vi "4Pi Quadrant Phase Extractor.vi"(7 "Calling VI Ref":refnum<vi>) -> ()   [LabVIEW 2016]
uses:
  <vilib>/vision/Image Controls.llb/IMAQ Image.ctl
  Hardware Configuration/Hardware Configuration Controls/Device Type.ctl
  Hardware Configuration/Hardware Configuration Controls/Device Function.ctl
  Device Library/Cameras/Hamamatsu/Orca Flash/Orca Flash Controls/Orca Flash Actions.ctl
  Device Library/Stages/Stages Controls/Stage Actions.ctl
  Device Library/Cameras/Camera Controls/Camera IMAQ Key Info.ctl
  Device Library/Stages/Stages Controls/Stage Status.ctl
  Display Module/Display Module Custom Controls/ROI Descriptor.ctl
  <vilib>/gmath/NumericalOptimization/Nonlinear Curve Fit LM formula string.vi
  <vilib>/Utility/file.llb/Write Delimited Spreadsheet (DBL).vi
  <vilib>/vision/NI_Vision_Development_Module.lvlib
  <resource>/objmgr/IMAQImage.rc
  <vilib>/gmath/NI_Gmath.lvlib
panel:
  in  "Overlay Plot":bool
  out "Overlay Plot Graph":cluster{dbl[], dbl[]}[](graph)
  in  "Z Stack":bool
  in  "Save Data":bool
  in  "Velocity (µm/s)":dbl
  in  "Position (µm)":dbl
  in  "Scan Range (µm)":dbl
  in  "Fit 04":bool
  in  "Fit 03":bool
  in  "Fit 02":bool
  in  "Fit 01":bool
  in  "Initial Guess Image 04":T1={"Offset"=100.0, "Amplitude"=50.0, "Wavelength"=15.0, "Phase"=1.0}
  in  "Initial Guess Image 03":T1={"Offset"=100.0, "Amplitude"=50.0, "Wavelength"=15.0, "Phase"=1.0}
  in  "Initial Guess Image 02":T1={"Offset"=100.0, "Amplitude"=50.0, "Wavelength"=15.0, "Phase"=1.0}
  in  "Initial Guess Image 01":T1={"Offset"=100.0, "Amplitude"=50.0, "Wavelength"=15.0, "Phase"=1.0}
  in  "Run Scan":bool
  out "ROI Plot 04":cluster{dbl[], dbl[]}[](graph)
  in  "Interference Image 04":i32(ring) items=["Quad 01", "Quad 02", "Quad 03", "Quad 04"]
  out "ROI Plot 03":cluster{dbl[], dbl[]}[](graph)
  in  "Interference Image 03":i32(ring) items=["Quad 01", "Quad 02", "Quad 03", "Quad 04"]
  out "ROI Plot 02":cluster{dbl[], dbl[]}[](graph)
  in  "Interference Image 02":i32(ring) items=["Quad 01", "Quad 02", "Quad 03", "Quad 04"]
  out "ROI Plot 01":cluster{dbl[], dbl[]}[](graph)
  in  "Interference Image 01":i32(ring) items=["Quad 01", "Quad 02", "Quad 03", "Quad 04"]
  in  "Quit":bool
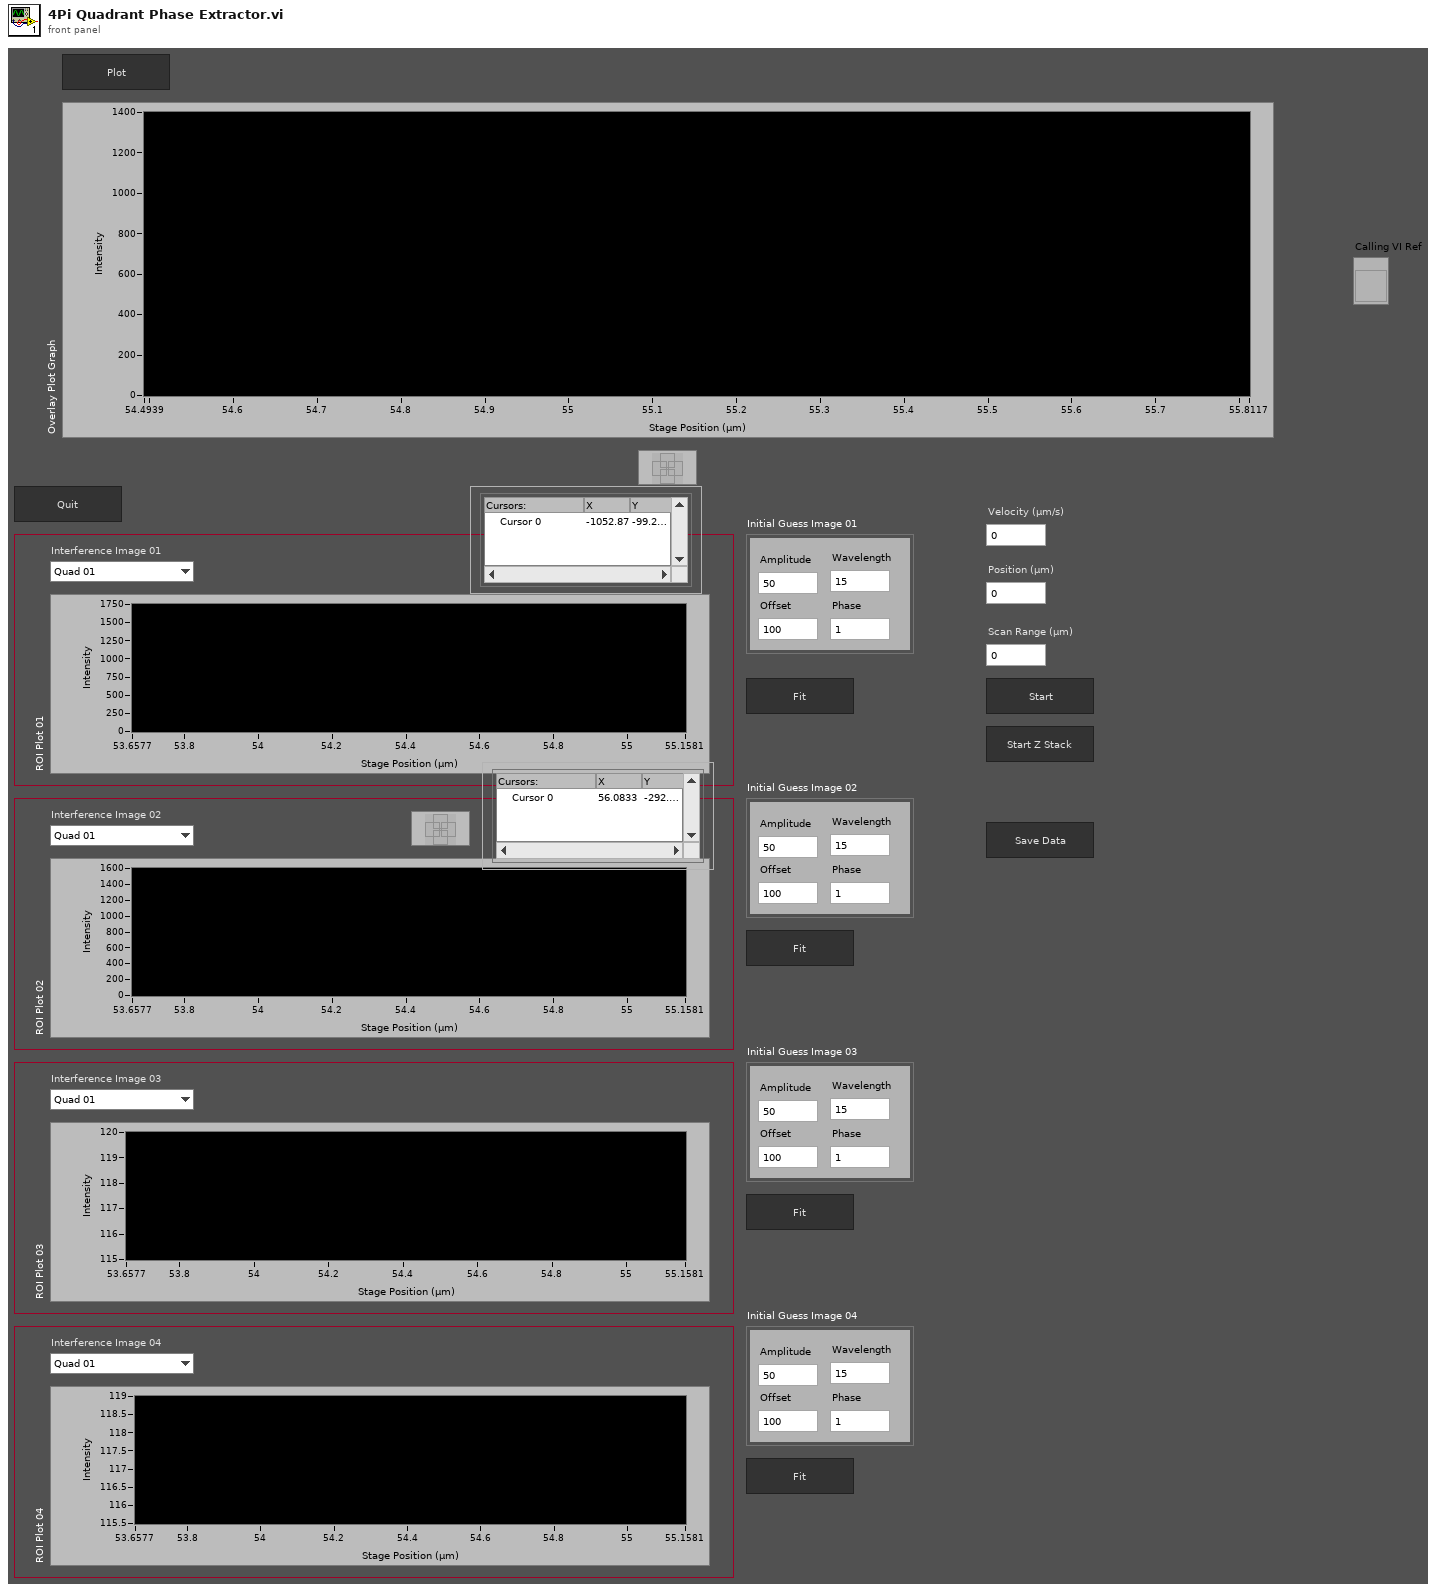
[diagram p1: front panel]
types:
  T1 = cluster{"Offset":dbl, "Amplitude":dbl, "Wavelength":dbl, "Phase":dbl}
  T2 = typedef "Device Function.ctl" = enum16{"Primary", "Secondary", "Overview", "Wide Field Drift Correction", "642 nm Excitation", "560 nm Excitation", "546 nm Excitation", "488 nm Excitation", "405 nm Excitation", "Objective Drift Correction", "Objective XY", "Objective Z", "Sample XY", "Sample Coarse Z", "Sample Z", "4Pi Lower", "4Pi Upper", "Adj Cavity"}
  T3 = typedef "Device Type.ctl" = enum16{"AOTF", "Camera", "Deformable Mirror", "Laser", "Shutter", "Stage"}
  T4 = typedef "Image Type" = u32
  T5 = typedef "Orca Flash Actions.ctl" = enum16{"IDLE", "PREVIEW", "RECORD", "Record Settings", "SETPARAM", "GETPARAM", "SETROI", "GETROI", "PROGRESSIVE MODE", "AREA MODE", "STATUS", "QUIT"}
  T6 = typedef "IMAQ Image.ctl" = refnum<image>
  T7 = typedef "Stage Actions.ctl" = enum16{"Get Position", "MVR", "MOVE", "HALT", "ONTARGET", "ERROR", "REFERENCE", "INIT", "VELOCITY", "STATUS", "EXIT", "HOME", "ZEROPOS", "NANOPOS", "ANALOG", "QUIT"}
  T8 = typedef "Camera IMAQ Key Info.ctl" = cluster{"Frame":u32, "Sensor Height":i32, "Sensor Width":i32, "ROI Height":i32, "ROI Width":i32, "ROI Enable?":bool, "Bit per Pixel":u8}
  T9 = typedef "Stage Status.ctl" = enum16{"Error", "Abort", "Busy", "On Target"}
  T10 = typedef "ROI Descriptor.ctl" = cluster{"Global Rectangle":i32[], "Contours":cluster{"Contour Type":u32, "ROI Type":u32, "Points":i32[]}[]}
  T11 = cluster{"model":string, "Parameters":string[], "x":string}
  T12 = cluster{"Mean Value":sgl, "Standard Variation":sgl, "Minimal Value":sgl, "Maximal Value":sgl, "Area (calibrated)":sgl, "Area (pixels)":u32, "%":sgl, "Calibration Valid":bool}
  T13 = cluster{"Numeric":dbl, "Numeric":dbl, "Numeric":dbl, "Numeric":dbl}
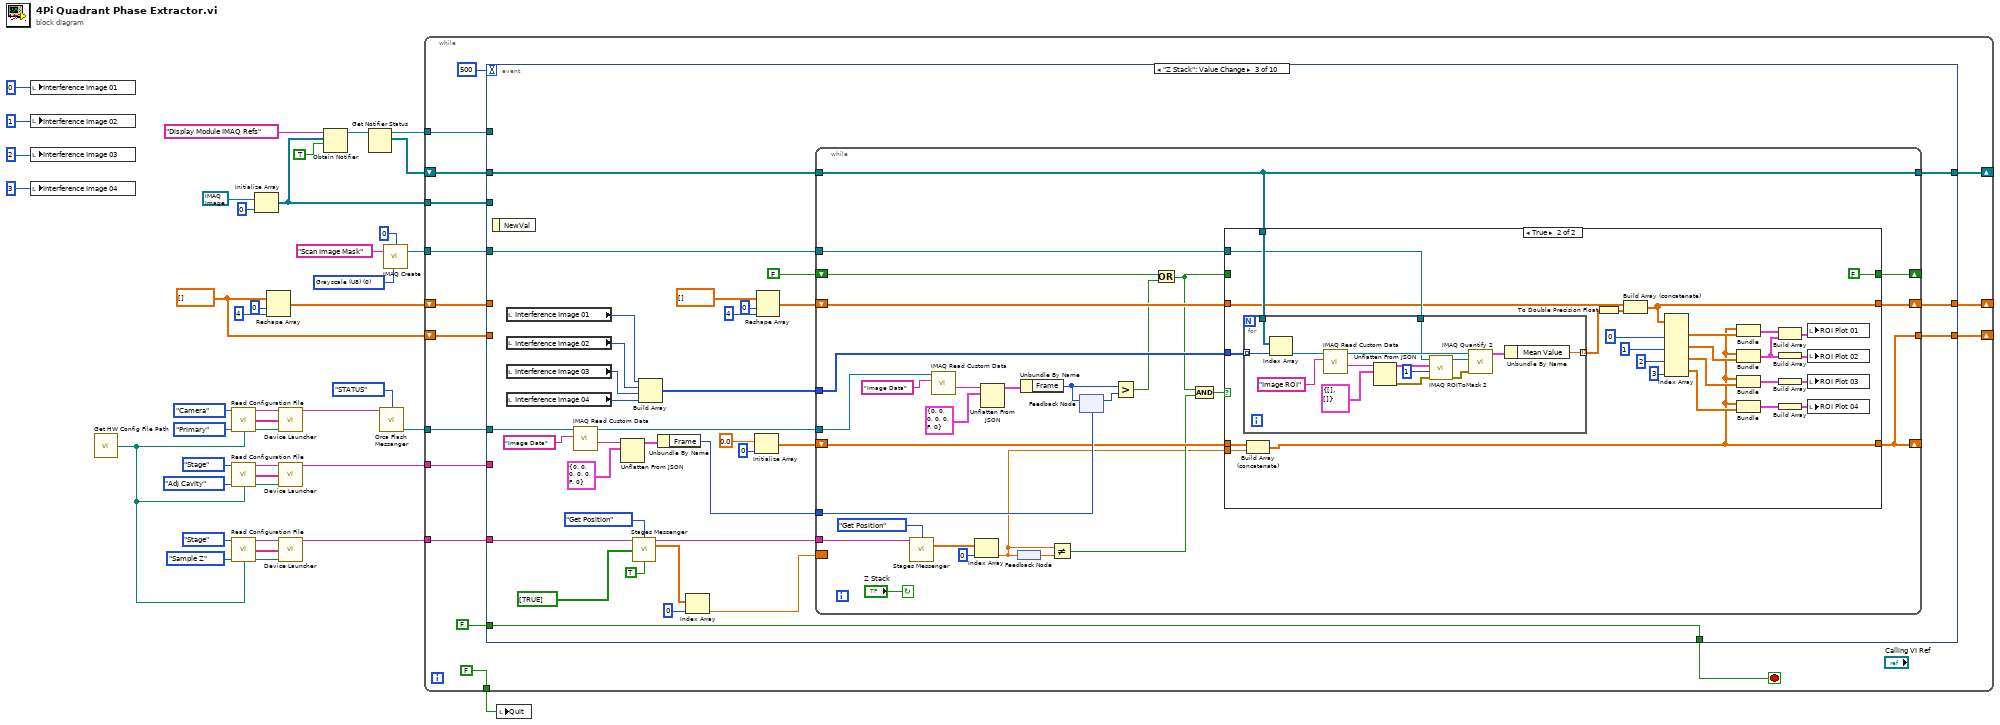
[diagram p0: block diagram]
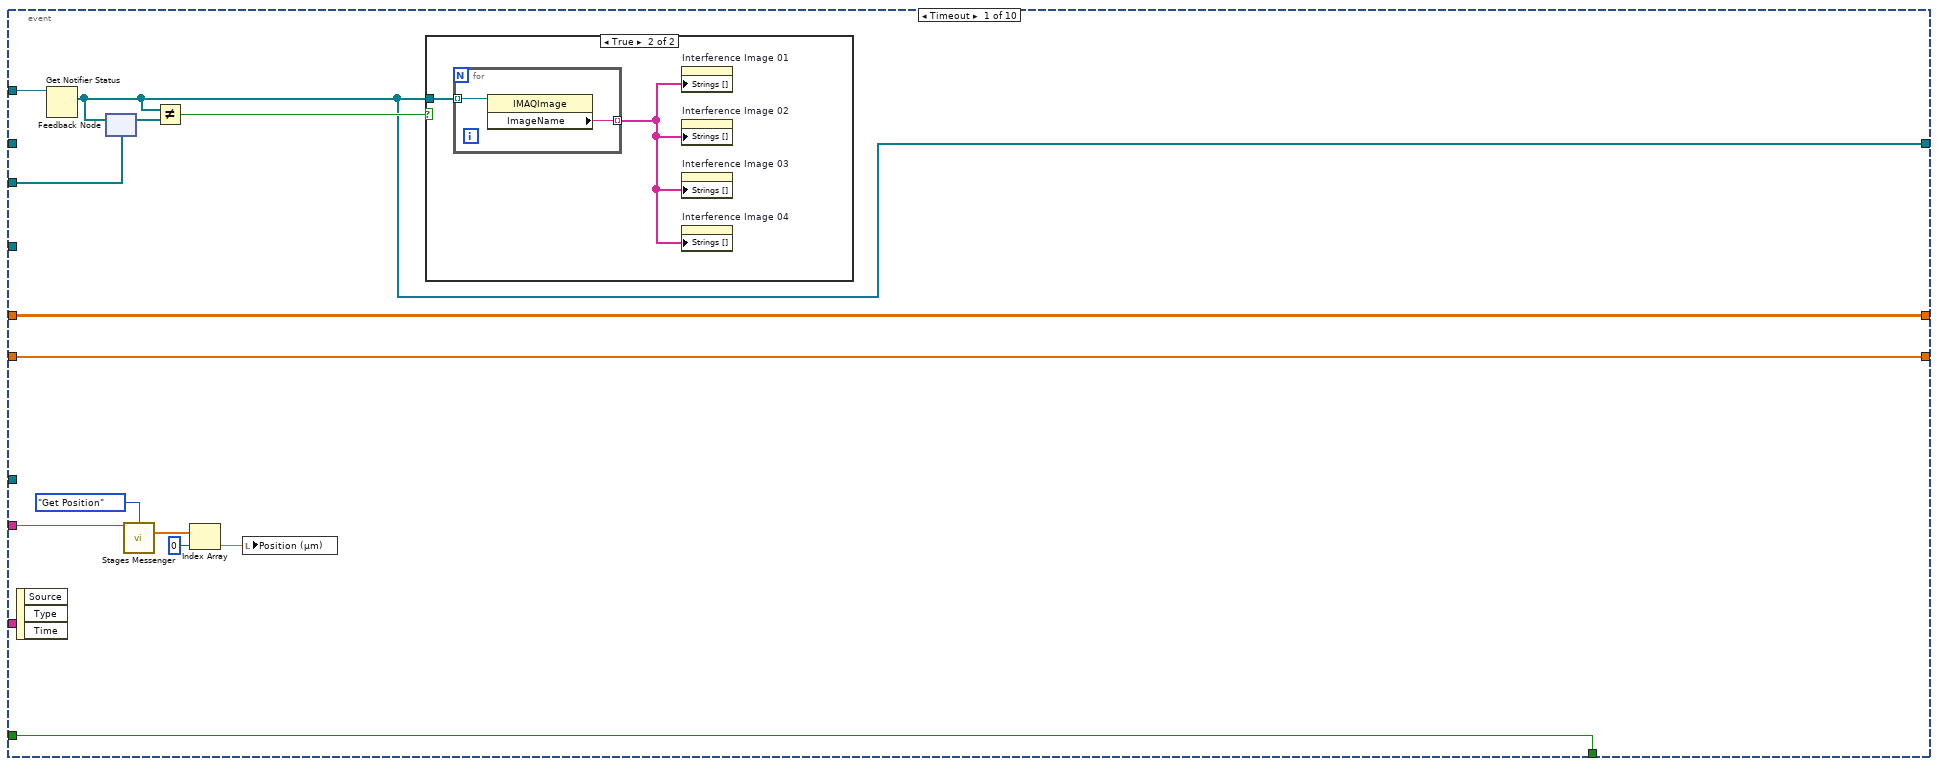
[diagram p2: hidden frame]
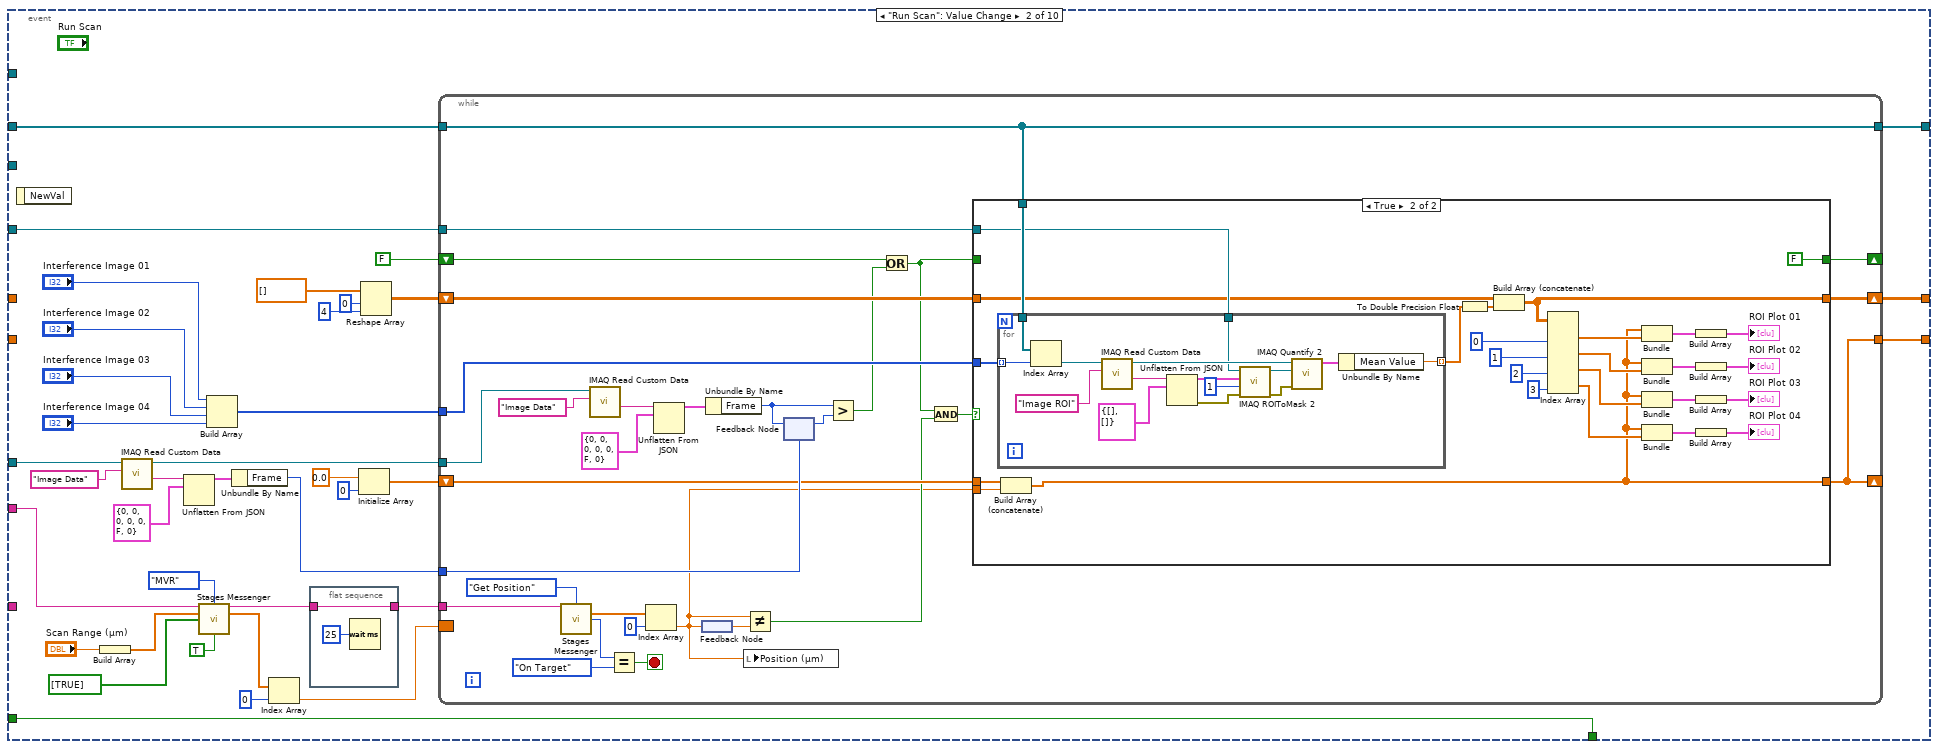
[diagram p4: hidden frame]
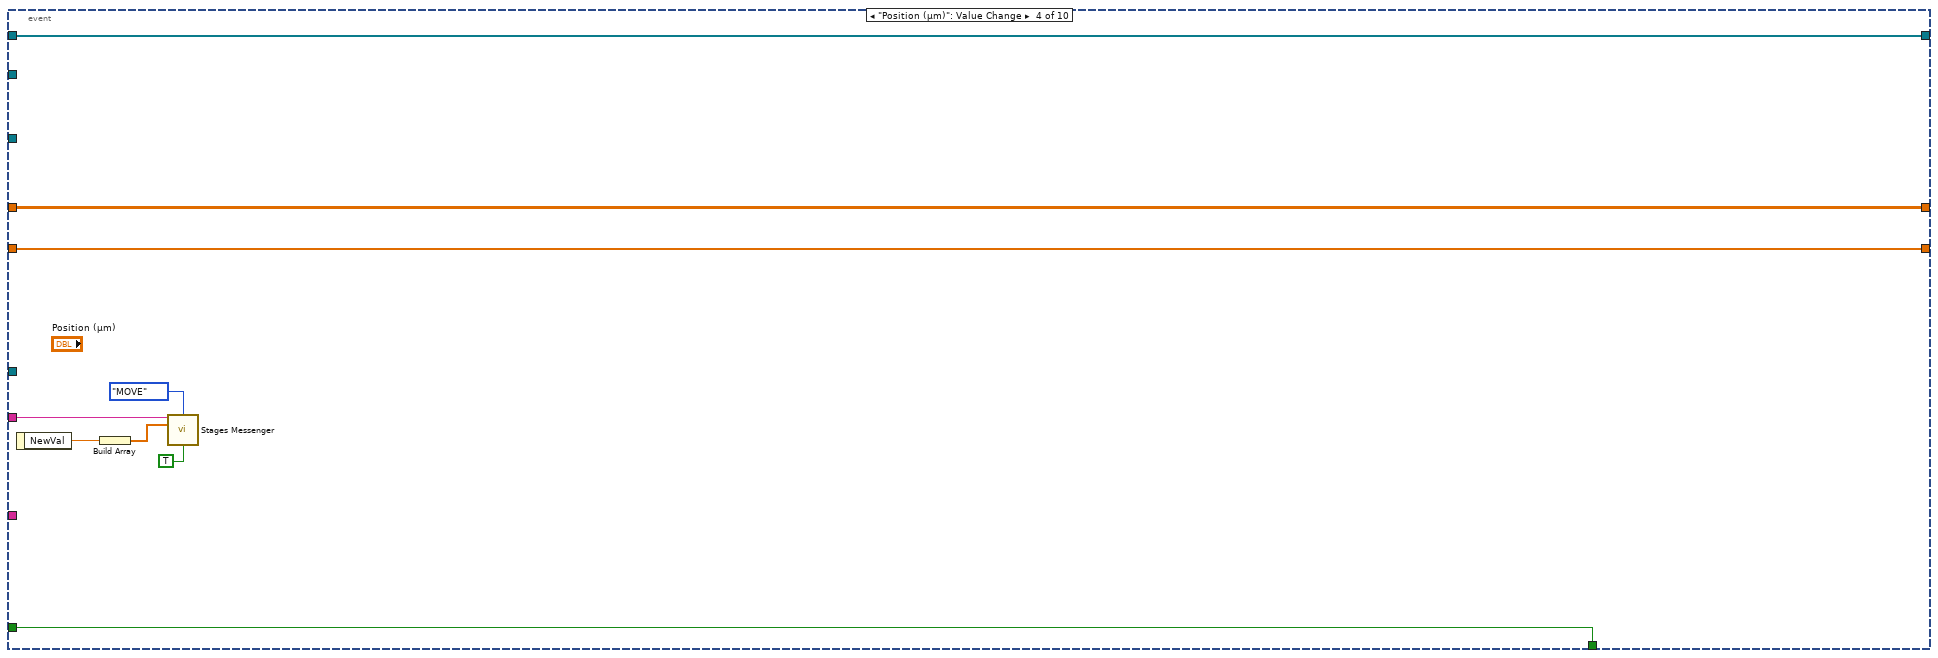
[diagram p7: hidden frame]
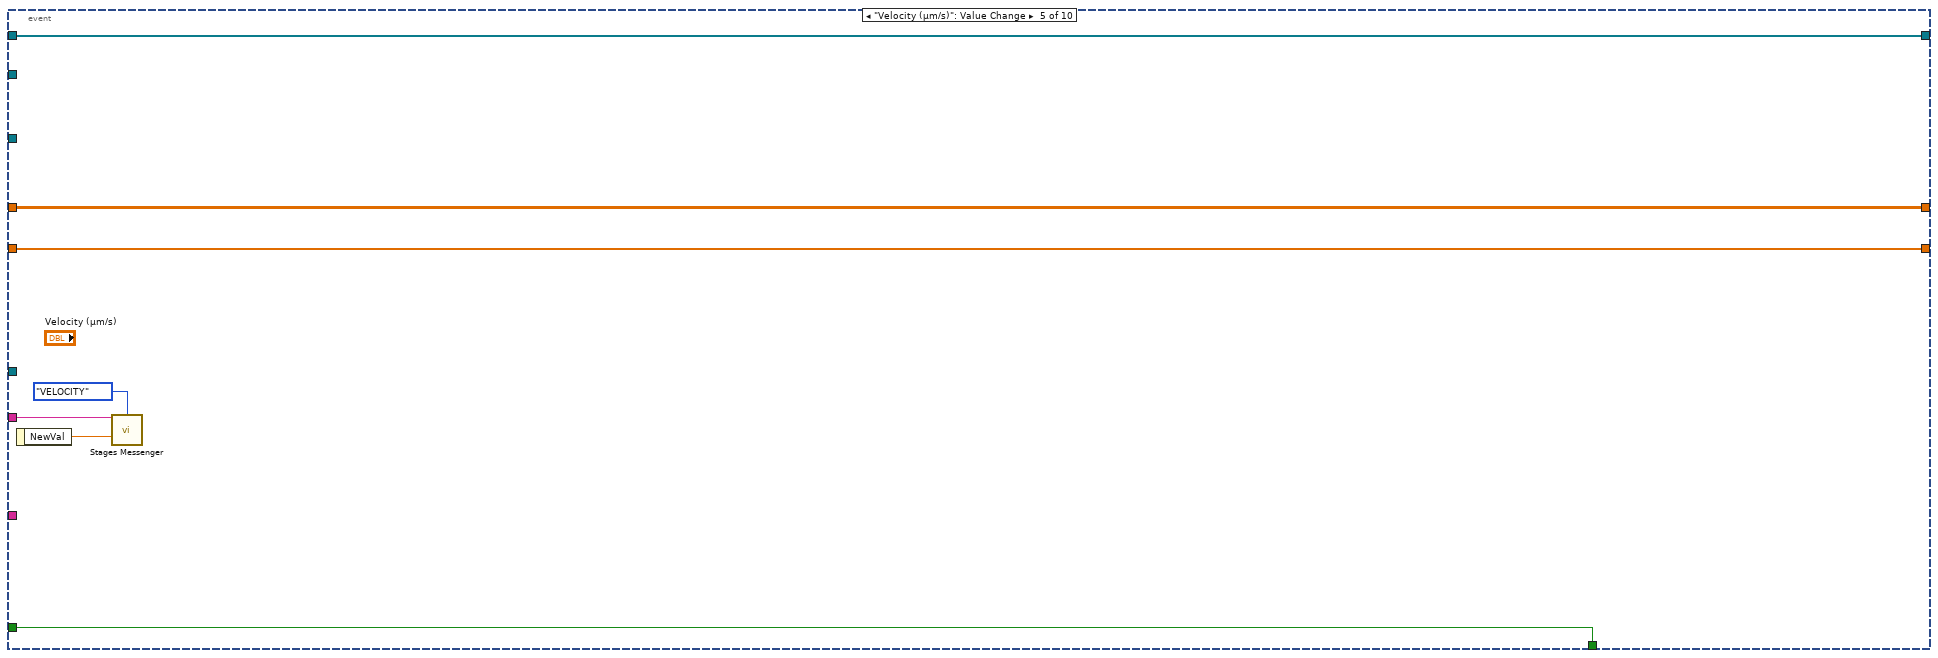
[diagram p8: hidden frame]
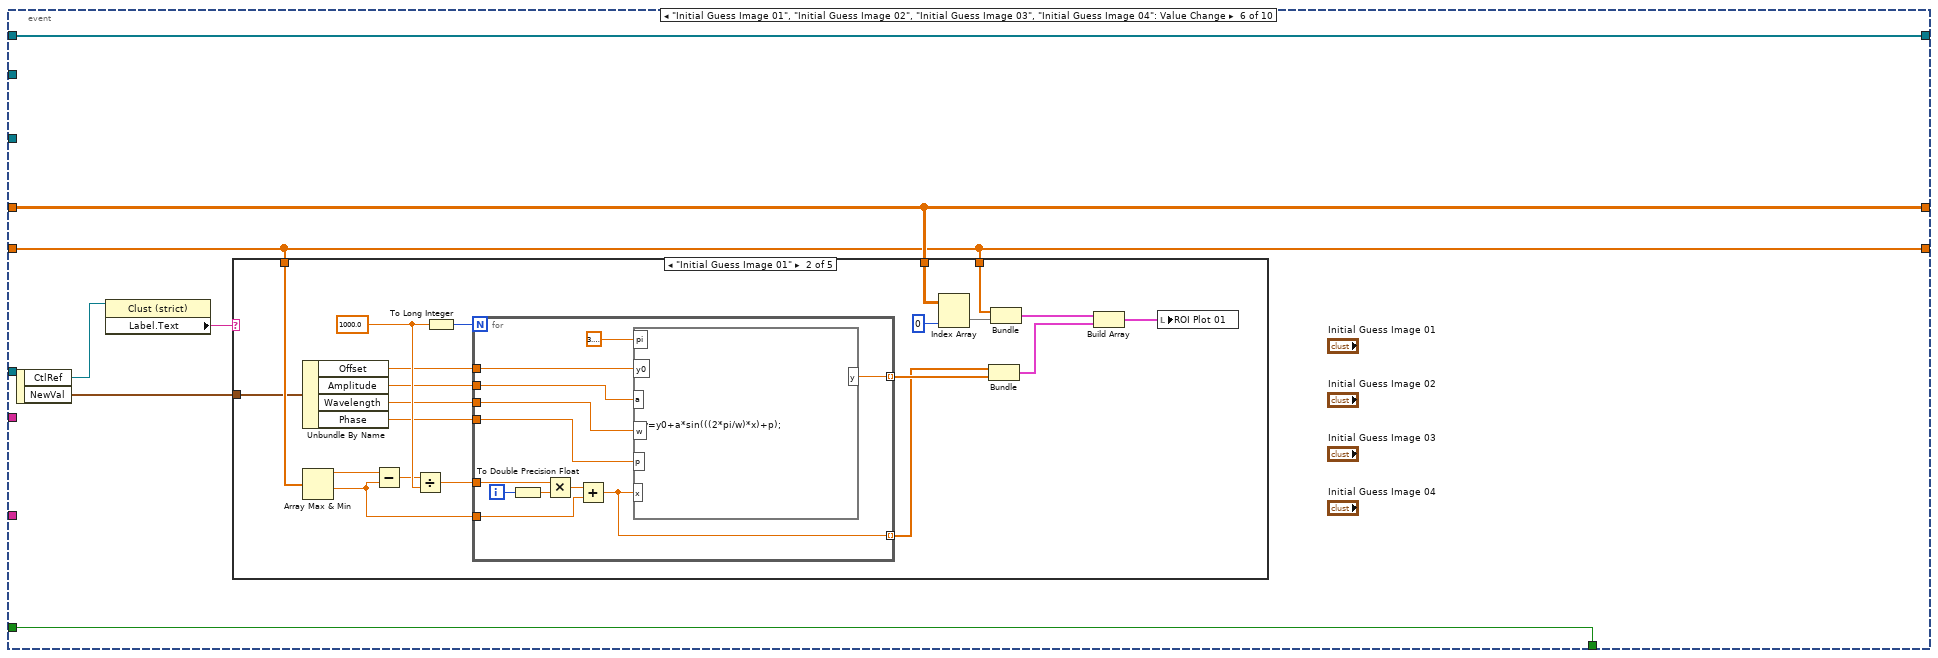
[diagram p9: hidden frame]
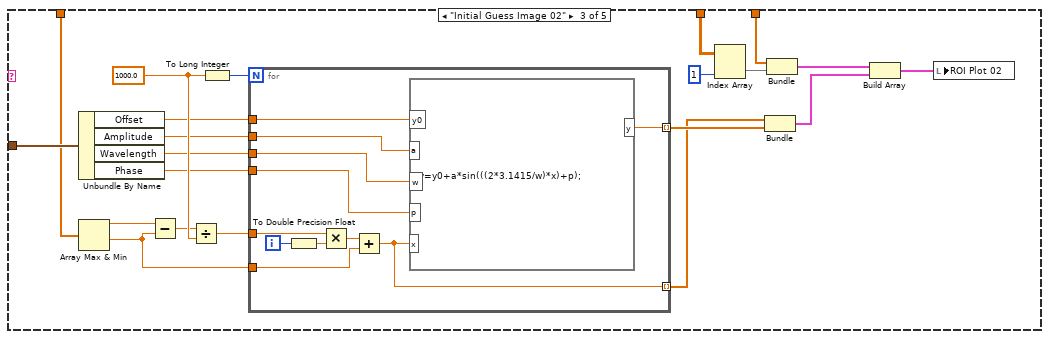
[diagram p11: hidden frame]
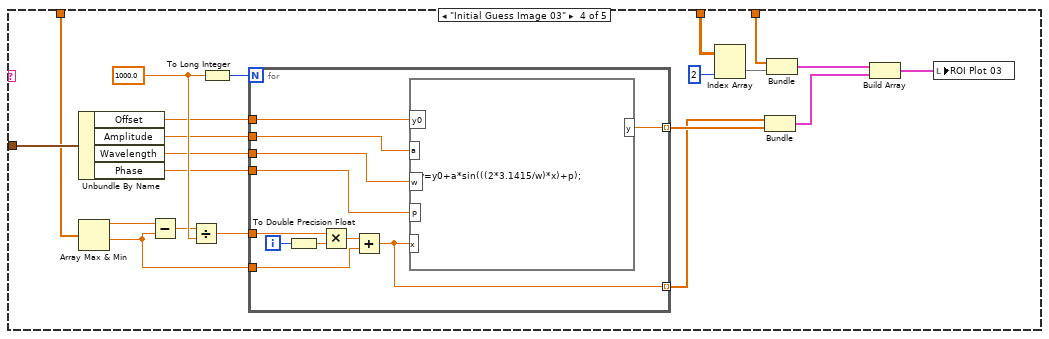
[diagram p12: hidden frame]
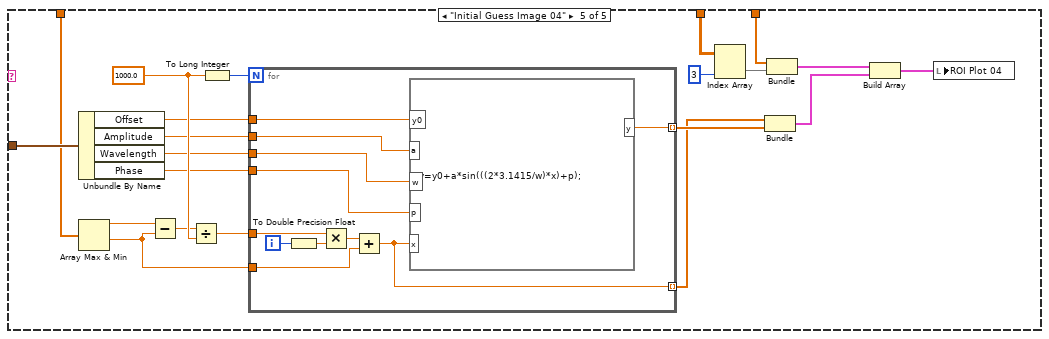
[diagram p13: hidden frame]
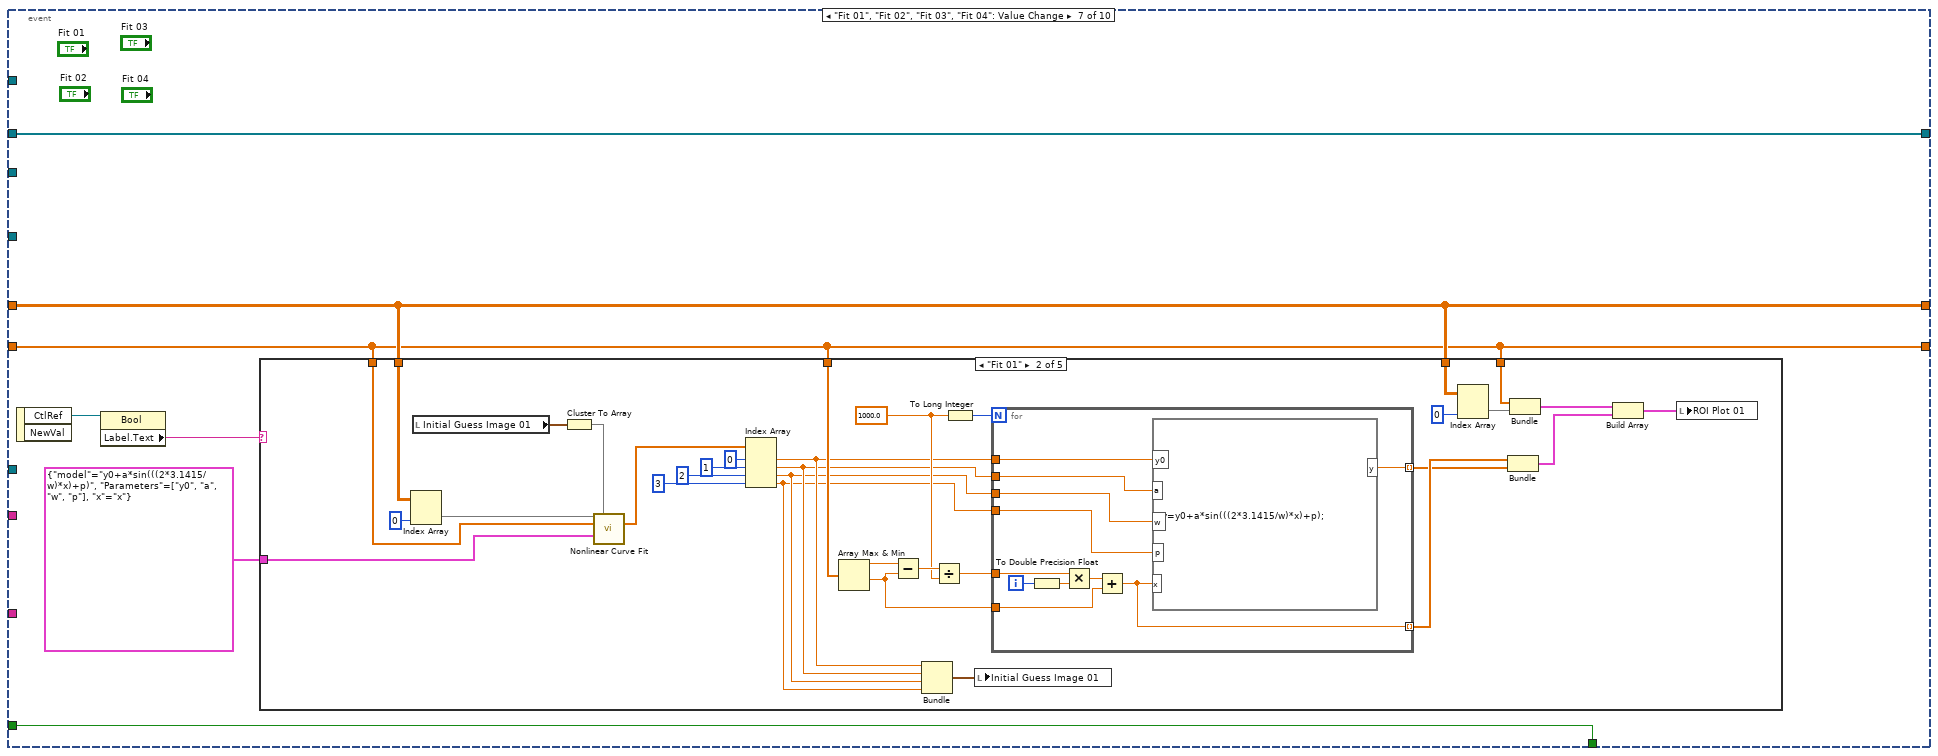
[diagram p14: hidden frame]
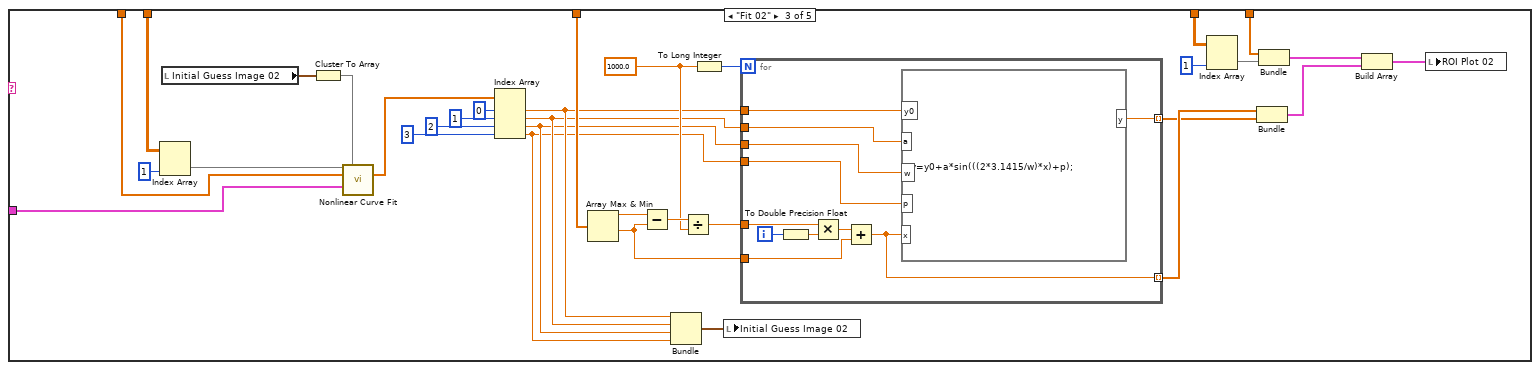
[diagram p16: hidden frame]
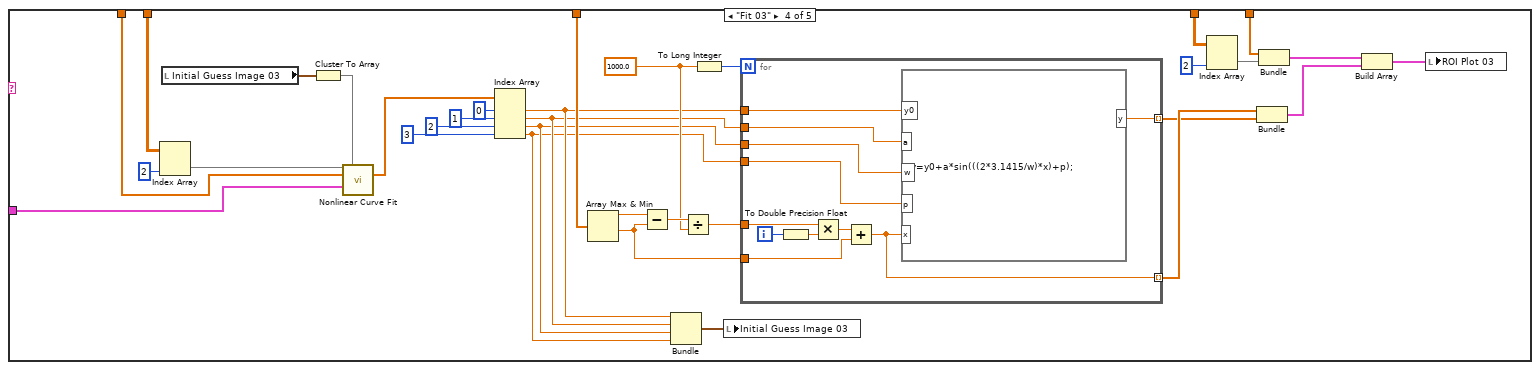
[diagram p17: hidden frame]
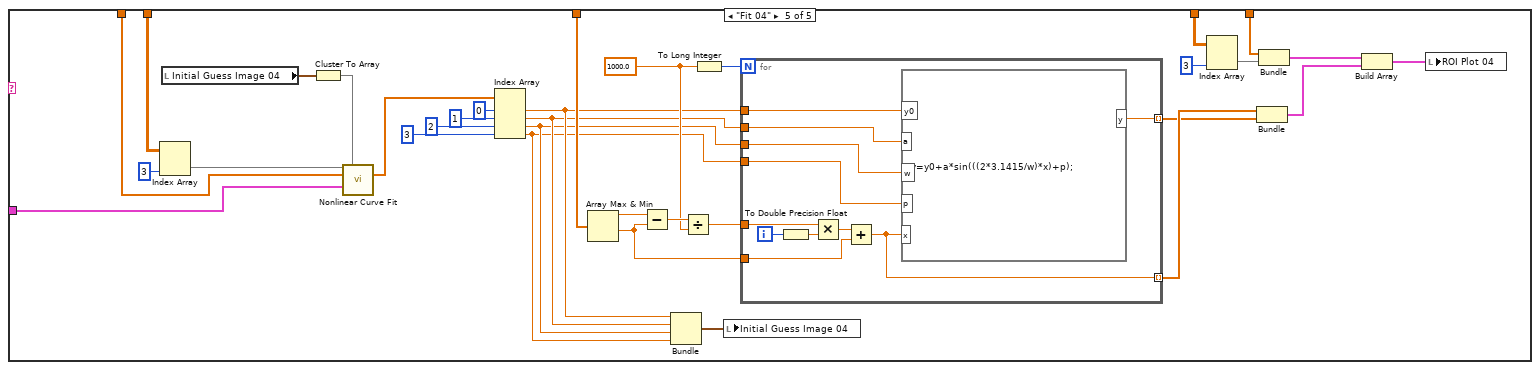
[diagram p18: hidden frame]
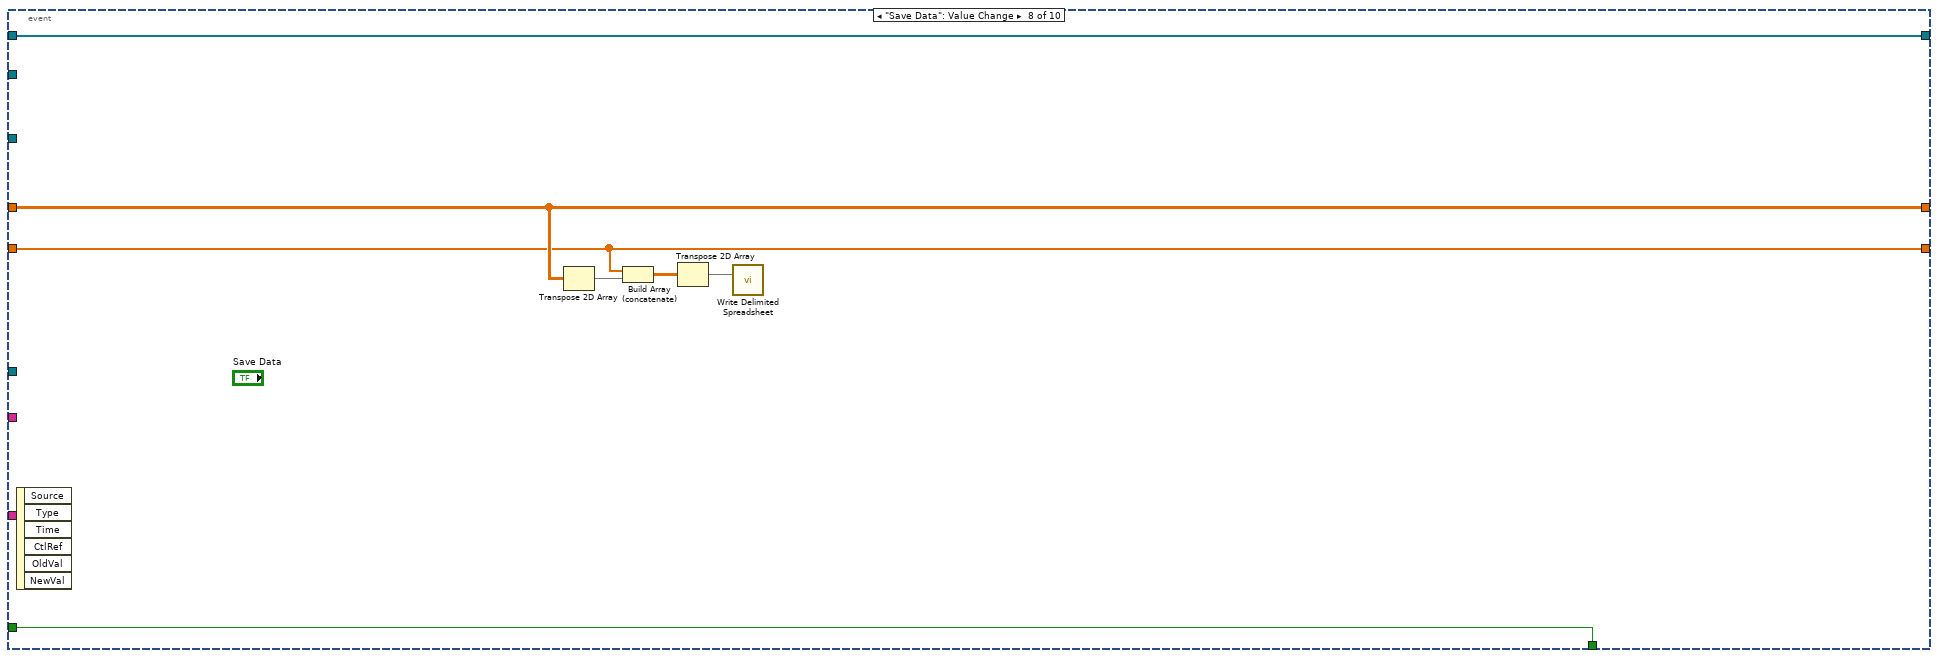
[diagram p19: hidden frame]
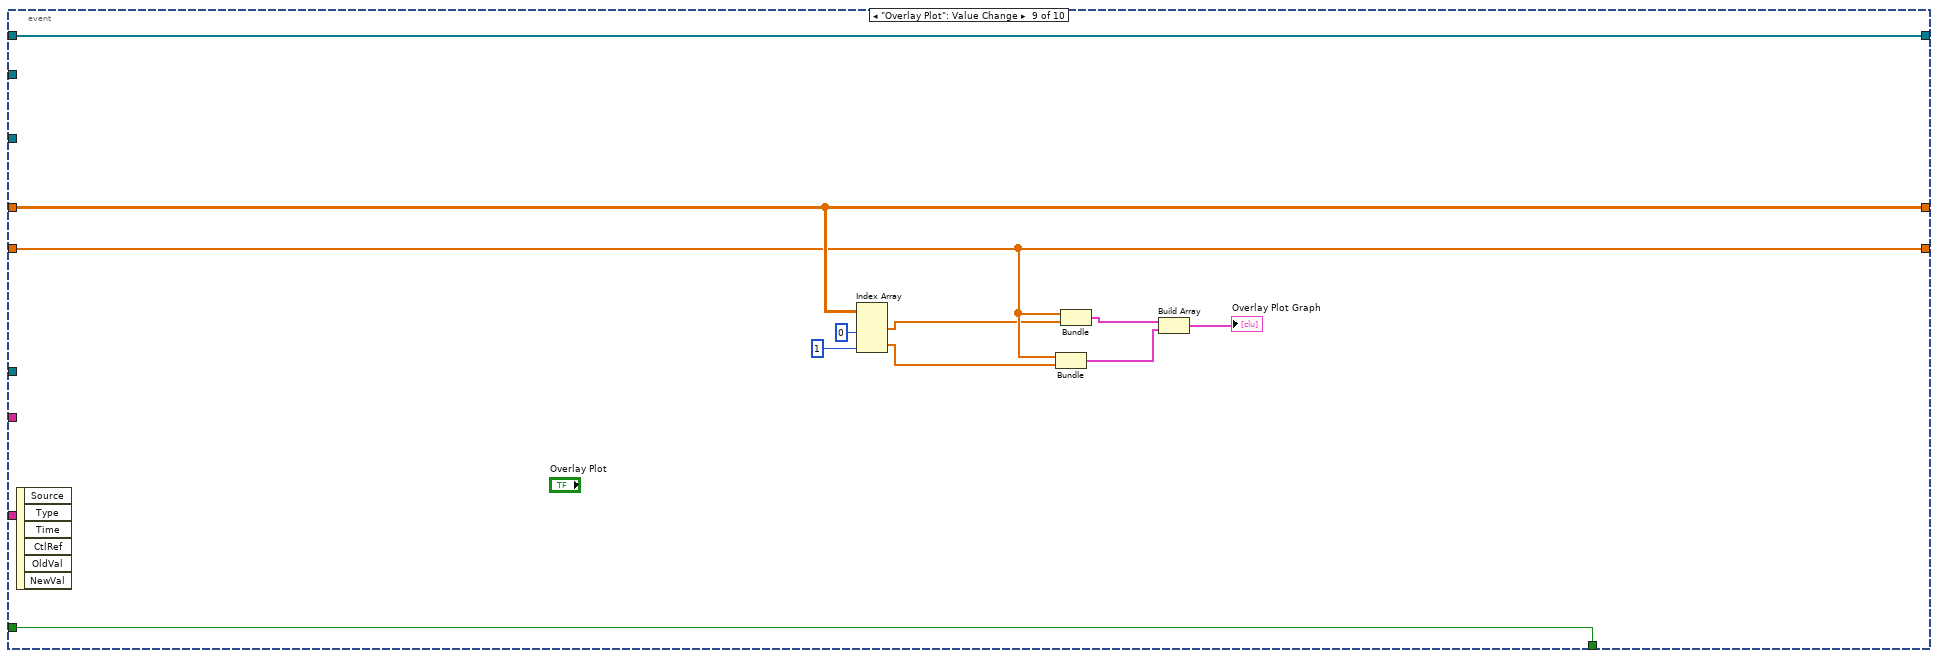
[diagram p20: hidden frame]
diagram:
  w18 = dbl[] [] ("array")
  w28 = T4 0 items=["Grayscale (U8)", "Grayscale (I16)", "Grayscale (SGL)", "Complex (CSG)", "RGB (U32)", "HSL (U32)", "RGB (U64)", "Grayscale (U16)"] ("Image Type")
  n1 = local write "Interference Image 01"(0) -> ()
  n2 = local write "Interference Image 02"(1) -> ()
  n3 = local write "Interference Image 03"(2) -> ()
  n4 = local write "Interference Image 04"(3) -> ()
  n5 = call "Get HW Config File Path.vi"() -> ("File Path"=w2:path)  [unwired: 14 in, 1 out]
  n6 = call "Read Configuration File.vi"("Device Type"=Device_Type."Camera", "Device Function"=Device_Function."Primary", "Config File Path"=w2) -> ("Unique Notifier Name"=w33:string, "Device Ports/IDs/Channels"=w35:string[], "Device Engine Path"=w34:path)  [unwired: 9 in, 1 out]
  n7 = call "Read Configuration File.vi"("Device Type"=Device_Type."Stage", "Device Function"=Device_Function."Adj Cavity", "Config File Path"=w2) -> ("Unique Notifier Name"=w9:string, "Device Ports/IDs/Channels"=w11:string[], "Device Engine Path"=w10:path)  [unwired: 9 in, 1 out]
  n8 = call "Read Configuration File.vi"("Device Type"=Device_Type."Stage", "Device Function"=Device_Function."Sample Z", "Config File Path"=w2) -> ("Unique Notifier Name"=w7:string, "Device Ports/IDs/Channels"=w5:string[], "Device Engine Path"=w6:path)  [unwired: 9 in, 1 out]
  n9 = Initialize Array(T6 refnum ("New Image"), 0 ("dimension size")) -> (w26:T6[])
  n10 = Reshape Array(w18, 0 ("dimension size"), 4 ("dimension size")) -> (w19:dbl[][])
  n11 = call "Device Launcher.vi"("Notifier Name"=w33, "Device Ports/IDs/Channels"=w35, "Device Engine Path"=w34) -> ("Notifier Name"=w31:string)  [unwired: 11 in, 1 out]
  n12 = call "Device Launcher.vi"("Notifier Name"=w9, "Device Ports/IDs/Channels"=w11, "Device Engine Path"=w10) -> ("Notifier Name"=w8:string)  [unwired: 11 in, 1 out]
  n13 = call "Device Launcher.vi"("Notifier Name"=w7, "Device Ports/IDs/Channels"=w5, "Device Engine Path"=w6) -> ("Notifier Name"=w1:string)  [unwired: 11 in, 1 out]
  n14 = Obtain Notifier(name (unnamed)="Display Module IMAQ Refs", notification data type=w26, create if not found? (T)=TRUE) -> (notifier out=w38:refnum<notifier>)  [unwired: 1 in, 2 out]
  n15 = Get Notifier Status(notifier=w38) -> (notifier out=w25:refnum<notifier>, current notification=w27:T6[])  [unwired: 1 in, 3 out]
  n16 = call "Orca Flash Messanger.vi"("Notifier Name"=w31, "Camera Actions"=Orca_Flash_Actions."STATUS") -> ("Image Ref"=w30:T6)  [unwired: 9 in, 4 out]
  n17 = call "IMAQ Create"("Border Size"=0, "Image Name"="Scan Image Mask", "Image Type"=w28) -> ("New Image"=w23:T6)  [unwired: 2 in, 1 out]
  n18 = while {
    tunnel: w30 -> [w51]
    tunnel: w26 -> [w56]
    tunnel: w25 -> [w55]
    tunnel: w23 -> [w54]
    shift-right: [w50] -> _
    shift-left: w27 -> [w57]
    tunnel: [FALSE] -> w22
    shift-right: [w48] -> _
    shift-left: w19 -> [w47]
    shift-right: [w45] -> _
    shift-left: w18 -> [w46]
    tunnel: w8 -> [w44]
    tunnel: w1 -> [w43]
    stop <- w53 stop-if-true
    n19 = event shown="[2] \"Z Stack\": Value Change" {
      selector: _ -> [_ _ _ _ _ _ _ _ _ _]
      dyn-events: _ -> [_ _ _ _ _ _ _ _ _ _]
      timeout: 500 -> [_ _ _ _ _ _ _ _ _ _]
      tunnel: w57 -> [_ w96 w211 w299 w309 w313 w449 w637 w649 w652]
      tunnel: w56 -> [w68 _ _ _ _ _ _ _ _ _]
      tunnel: w55 -> [w69 _ _ _ _ _ _ _ _ w655]
      tunnel: w54 -> [_ w95 w210 _ _ _ _ _ _ w654]
      tunnel: [w67 w112 w223 w300 w310 w319 w455 w638 w648 w653] -> w53
      tunnel: FALSE -> [w67 w112 w223 w300 w310 w319 w455 w638 w648 _]
      tunnel: w51 -> [_ w108 w219 _ _ _ _ _ _ _]
      tunnel: [w66 w92 w207 w299 w309 w313 w449 w637 w649 w652] -> w50
      tunnel: [w65 w91 w206 w298 w308 w317 w451 w636 w647 w651] -> w48
      tunnel: w47 -> [w65 _ _ w298 w308 w317 w451 w636 w647 w651]
      tunnel: w46 -> [w64 _ _ w297 w307 w315 w450 w634 w644 w650]
      tunnel: [w64 w90 w205 w297 w307 w315 w450 w634 w644 w650] -> w45
      tunnel: w44 -> [w63 w82 _ w303 w311 _ _ _ _ _]
      tunnel: w43 -> [_ _ w194 _ _ _ _ _ _ _]
      event Timeout {
        n20 = event-data() -> ()  [unwired: 1 in, 3 out]
        n21 = Get Notifier Status(notifier=w69) -> (current notification=w66:T6[])  [unwired: 1 in, 4 out]
        n22 = feedback #1(w68) -> (w70:T6[])
        n23 = feedback-in #1(w66) -> ()
        n24 = call "Stages Messenger.vi"("Stage Notifier Name"=w63, "Actions"=Stage_Actions."Get Position") -> ("Positions"=w61:dbl[])  [unwired: 10 in, 3 out]
        n25 = Not Equal?(x=w66, y=w70) -> (x != y?=w71:bool)
        n26 = Index Array(array=w61, index=0) -> (element=w59:dbl)
        n27 = local write "Position (µm)"(w59) -> ()
        n28 = case shown="True" w71 {
          tunnel: w66 -> [_ w73]
          frame False {
          }
          frame True {
            n29 = for {
              tunnel: w73 -> [w75] mode=indexing
              tunnel: [w74] -> w72 mode=indexing
              n30 = property class="IMAQImage"(reference=w75) -> ("ImageName"=w74:string)  [unwired: 1 in, 2 out]
            }
            n31 = property on="Interference Image 01" class="Ring (strict)"("Strings []"=w72) -> ()  [unwired: 2 in, 2 out]
            n32 = property on="Interference Image 02" class="Ring (strict)"("Strings []"=w72) -> ()  [unwired: 2 in, 2 out]
            n33 = property on="Interference Image 03" class="Ring (strict)"("Strings []"=w72) -> ()  [unwired: 2 in, 2 out]
            n34 = property on="Interference Image 04" class="Ring (strict)"("Strings []"=w72) -> ()  [unwired: 2 in, 2 out]
          }
        }
      }
      event "Run Scan": Value Change {
        n35 = event-data() -> ()  [unwired: 1 in, 1 out]
        n36 = Build Array("Scan Range (µm)") -> (w85:dbl[])
        n37 = call "IMAQ Read Custom Data"("Key"="Image Data", "Image"=w108) -> ("Custom Data Out"=w110:string, "Image (duplicate)"=w107:T6)  [unwired: 7 in, 1 out]
        n38 = Unflatten From JSON(JSON string=w110, type and defaults=T8 {"Frame"=0, "Sensor Height"=0, "Sensor Width"=0, "ROI Height"=0, "ROI Width"=0, "ROI Enable?"=FALSE, "Bit per Pixel"=0} ("Camera IMAQ Key Info")) -> (value=w106:T8)  [unwired: 5 in, 1 out]
        n39 = call "Stages Messenger.vi"("Stage Notifier Name"=w82, "Actions"=Stage_Actions."MVR", "Setpoint"=w85, "Axis"=bool[] [TRUE], "Exit While Busy?"=TRUE) -> ("Stage Notifier Name (Dup)"=w77:string, "Positions"=w81:dbl[])  [unwired: 7 in, 2 out]
        n40 = Build Array("Interference Image 01", "Interference Image 02", "Interference Image 03", "Interference Image 04") -> (w94:i32[])
        n41 = Unbundle By Name(w106) -> ("Frame"=w93:u32)
        n42 = Index Array(array=w81, index=0) -> (element=w79:dbl)
        n43 = flat-sequence {
          tunnel: w77 -> [w114]
          tunnel: [w114] -> w76
          frame #0 {
            n44 = Wait (ms)(milliseconds to wait=u32 25) -> ()  [unwired: 1 out]
          }
        }
        n45 = Initialize Array(0.0 ("element"), 0 ("dimension size")) -> (w104:dbl[])
        n46 = Reshape Array(sgl[] [] ("array"), 0 ("dimension size"), 4 ("dimension size")) -> (w97:sgl[][])
        n47 = while {
          tunnel: w107 -> [w135]
          shift-right: [w119] -> _
          shift-left: w104 -> [w133]
          shift-right: [w141] -> w91
          shift-left: w97 -> [w142]
          tunnel: w96 -> [w131]
          tunnel: w95 -> [w144]
          tunnel: w94 -> [w143]
          tunnel: w93 -> [w134]
          tunnel: [w131] -> w92
          tunnel: [w119] -> w90
          tunnel: w76 -> [w127]
          border: w79 -> [_]
          shift-right: [w116] -> _
          shift-left: FALSE -> [w120]
          stop <- w128 stop-if-true
          n48 = call "Stages Messenger.vi"("Stage Notifier Name"=w127, "Actions"=Stage_Actions."Get Position") -> ("Positions"=w126:dbl[], "Status"=w130:T9)  [unwired: 10 in, 2 out]
          n49 = call "IMAQ Read Custom Data"("Key"="Image Data", "Image"=w135) -> ("Custom Data Out"=w137:string)  [unwired: 7 in, 2 out]
          n50 = Equal?(x=w130, y=Stage_Status."On Target") -> (x = y?=w128:bool)
          n51 = Index Array(array=w126, index=0) -> (element=w115:dbl)
          n52 = Unflatten From JSON(JSON string=w137, type and defaults=T8 {"Frame"=0, "Sensor Height"=0, "Sensor Width"=0, "ROI Height"=0, "ROI Width"=0, "ROI Enable?"=FALSE, "Bit per Pixel"=0} ("Camera IMAQ Key Info")) -> (value=w139:T8)  [unwired: 5 in, 1 out]
          n53 = feedback-in #2(w115) -> ()
          n54 = feedback #2() -> (w124:dbl)
          n55 = Unbundle By Name(w139) -> ("Frame"=w132:u32)
          n56 = local write "Position (µm)"(w115) -> ()
          n57 = Not Equal?(x=w115, y=w124) -> (x != y?=w123:bool)
          n58 = feedback #3(w134) -> (w140:u32)
          n59 = feedback-in #3(w132) -> ()
          n60 = Greater?(x=w132, y=w140) -> (0:w118:bool)
          n61 = Or(x=w120, y=w118) -> (x .or. y?=w117:bool)
          n62 = And(x=w117, y=w123) -> (x .and. y?=w122:bool)
          n63 = case shown="True" w122 {
            tunnel: w131 -> [_ w174]
            tunnel: w144 -> [_ w173]
            tunnel: w143 -> [_ w172]
            tunnel: w142 -> [w147 w171]
            tunnel: [w147 w167] -> w141
            tunnel: w133 -> [w146 w169]
            tunnel: [w146 w156] -> w119
            tunnel: w115 -> [_ w168]
            tunnel: w117 -> [w145 _]
            tunnel: [w145 FALSE] -> w116
            frame False {
            }
            frame True {
              n64 = for {
                tunnel: w172 -> [w180] mode=indexing
                tunnel: [w177] -> w170 mode=indexing
                tunnel: w174 -> [w176]
                tunnel: w173 -> [w175]
                n65 = Index Array(array=w176, index=w180) -> (element=w178:T6)
                n66 = call "IMAQ Read Custom Data"("Key"="Image ROI", "Image"=w178) -> ("Custom Data Out"=w188:string, "Image (duplicate)"=w181:T6)  [unwired: 7 in, 1 out]
                n67 = Unflatten From JSON(JSON string=w188, type and defaults=T10 {"Global Rectangle"=[], "Contours"=[]} ("Image ROI Descriptor")) -> (value=w187:T10, error out=w183:errorcluster)  [unwired: 5 in]
                n68 = call "IMAQ ROIToMask 2"("error in (no error)"=w183, "Filling Value (255)"=1, "ROI Descriptor"=w187, "Image"=w175) -> ("error out"=w184:errorcluster, "Image Out"=w185:T6)  [unwired: 5 in, 1 out]
                n69 = call "IMAQ Quantify 2"("error in (no error)"=w184, "Image Mask"=w185, "Image"=w181) -> ("Global Report"=w182:T12)  [unwired: 6 in, 2 out]
                n70 = Unbundle By Name(w182) -> ("Mean Value"=w177:sgl)
              }
              n71 = Build Array (concatenate)(w169, w168) -> (w156:dbl[])
              n72 = To Double Precision Float(number=w170) -> (double precision float=w149:dbl[])
              n73 = Build Array (concatenate)(w171, w149) -> (w167:dbl[][])
              n74 = Index Array(array=w167, index (col) #1=0 ("disabled index (col)"), index (col) #2=1 ("index (col)"), index (col) #3=2 ("index (col)"), index (col) #4=3 ("index (col)")) -> (element #1=w162:dbl[], element #2=w161:dbl[], element #3=w160:dbl[], element #4=w159:dbl[])  [unwired: 4 in]
              n75 = Bundle(w156, w162) -> (w158:cluster{dbl[], dbl[]})  [unwired: 1 in]
              n76 = Bundle(w156, w161) -> (w155:cluster{dbl[], dbl[]})  [unwired: 1 in]
              n77 = Bundle(w156, w160) -> (w154:cluster{dbl[], dbl[]})  [unwired: 1 in]
              n78 = Bundle(w156, w159) -> (w153:cluster{dbl[], dbl[]})  [unwired: 1 in]
              n79 = Build Array(w158) -> (→"ROI Plot 01":cluster{dbl[], dbl[]}[])
              n80 = Build Array(w155) -> (→"ROI Plot 02":cluster{dbl[], dbl[]}[])
              n81 = Build Array(w154) -> (→"ROI Plot 03":cluster{dbl[], dbl[]}[])
              n82 = Build Array(w153) -> (→"ROI Plot 04":cluster{dbl[], dbl[]}[])
            }
          }
        }
      }
      event "Z Stack": Value Change {
        n83 = event-data() -> ()  [unwired: 1 in, 1 out]
        n84 = local read "Interference Image 01"() -> (w190:i32)
        n85 = local read "Interference Image 02"() -> (w191:i32)
        n86 = local read "Interference Image 03"() -> (w192:i32)
        n87 = local read "Interference Image 04"() -> (w193:i32)
        n88 = call "IMAQ Read Custom Data"("Key"="Image Data", "Image"=w219) -> ("Custom Data Out"=w221:string, "Image (duplicate)"=w218:T6)  [unwired: 7 in, 1 out]
        n89 = Unflatten From JSON(JSON string=w221, type and defaults=T8 {"Frame"=0, "Sensor Height"=0, "Sensor Width"=0, "ROI Height"=0, "ROI Width"=0, "ROI Enable?"=FALSE, "Bit per Pixel"=0} ("Camera IMAQ Key Info")) -> (value=w217:T8)  [unwired: 5 in, 1 out]
        n90 = call "Stages Messenger.vi"("Stage Notifier Name"=w194, "Actions"=Stage_Actions."Get Position", "Axis"=bool[] [TRUE], "Exit While Busy?"=TRUE) -> ("Stage Notifier Name (Dup)"=w195:string, "Positions"=w199:dbl[])  [unwired: 8 in, 2 out]
        n91 = Build Array(w190, w191, w192, w193) -> (w209:i32[])
        n92 = Unbundle By Name(w217) -> ("Frame"=w208:u32)
        n93 = Index Array(array=w199, index=0) -> (element=w197:dbl)
        n94 = Initialize Array(0.0 ("element"), 0 ("dimension size")) -> (w215:dbl[])
        n95 = Reshape Array(sgl[] [] ("array"), 0 ("dimension size"), 4 ("dimension size")) -> (w212:sgl[][])
        n96 = while {
          tunnel: w218 -> [w242]
          shift-right: [w229] -> _
          shift-left: w215 -> [w240]
          shift-right: [w248] -> w206
          shift-left: w212 -> [w249]
          tunnel: w211 -> [w238]
          tunnel: w210 -> [w251]
          tunnel: w209 -> [w250]
          tunnel: w208 -> [w241]
          tunnel: [w238] -> w207
          tunnel: [w229] -> w205
          tunnel: w195 -> [w237]
          border: w197 -> [_]
          shift-right: [w226] -> _
          shift-left: FALSE -> [w230]
          stop <- "Z Stack" continue-if-true
          n97 = call "Stages Messenger.vi"("Stage Notifier Name"=w237, "Actions"=Stage_Actions."Get Position") -> ("Positions"=w236:dbl[])  [unwired: 10 in, 3 out]
          n98 = call "IMAQ Read Custom Data"("Key"="Image Data", "Image"=w242) -> ("Custom Data Out"=w244:string)  [unwired: 7 in, 2 out]
          n99 = Index Array(array=w236, index=0) -> (element=w225:dbl)
          n100 = Unflatten From JSON(JSON string=w244, type and defaults=T8 {"Frame"=0, "Sensor Height"=0, "Sensor Width"=0, "ROI Height"=0, "ROI Width"=0, "ROI Enable?"=FALSE, "Bit per Pixel"=0} ("Camera IMAQ Key Info")) -> (value=w246:T8)  [unwired: 5 in, 1 out]
          n101 = feedback-in #4(w225) -> ()
          n102 = feedback #4() -> (w234:dbl)
          n103 = Unbundle By Name(w246) -> ("Frame"=w239:u32)
          n104 = Not Equal?(x=w225, y=w234) -> (x != y?=w233:bool)
          n105 = feedback #5(w241) -> (w247:u32)
          n106 = feedback-in #5(w239) -> ()
          n107 = Greater?(x=w239, y=w247) -> (0:w228:bool)
          n108 = Or(x=w230, y=w228) -> (x .or. y?=w227:bool)
          n109 = And(x=w227, y=w233) -> (x .and. y?=w232:bool)
          n110 = case shown="True" w232 {
            tunnel: w238 -> [_ w281]
            tunnel: w251 -> [_ w280]
            tunnel: w250 -> [_ w279]
            tunnel: w249 -> [w254 w278]
            tunnel: [w254 w274] -> w248
            tunnel: w240 -> [w253 w276]
            tunnel: [w253 w264] -> w229
            tunnel: w225 -> [_ w275]
            tunnel: w227 -> [w252 _]
            tunnel: [w252 FALSE] -> w226
            frame False {
            }
            frame True {
              n111 = for {
                tunnel: w279 -> [w287] mode=indexing
                tunnel: [w284] -> w277 mode=indexing
                tunnel: w281 -> [w283]
                tunnel: w280 -> [w282]
                n112 = Index Array(array=w283, index=w287) -> (element=w285:T6)
                n113 = call "IMAQ Read Custom Data"("Key"="Image ROI", "Image"=w285) -> ("Custom Data Out"=w295:string, "Image (duplicate)"=w288:T6)  [unwired: 7 in, 1 out]
                n114 = Unflatten From JSON(JSON string=w295, type and defaults=T10 {"Global Rectangle"=[], "Contours"=[]} ("Image ROI Descriptor")) -> (value=w294:T10, error out=w290:errorcluster)  [unwired: 5 in]
                n115 = call "IMAQ ROIToMask 2"("error in (no error)"=w290, "Filling Value (255)"=1, "ROI Descriptor"=w294, "Image"=w282) -> ("error out"=w291:errorcluster, "Image Out"=w292:T6)  [unwired: 5 in, 1 out]
                n116 = call "IMAQ Quantify 2"("error in (no error)"=w291, "Image Mask"=w292, "Image"=w288) -> ("Global Report"=w289:T12)  [unwired: 6 in, 2 out]
                n117 = Unbundle By Name(w289) -> ("Mean Value"=w284:sgl)
              }
              n118 = Build Array (concatenate)(w276, w275) -> (w264:dbl[])
              n119 = To Double Precision Float(number=w277) -> (double precision float=w261:dbl[])
              n120 = Build Array (concatenate)(w278, w261) -> (w274:dbl[][])
              n121 = Index Array(array=w274, index (col) #1=0 ("disabled index (col)"), index (col) #2=1 ("index (col)"), index (col) #3=2 ("index (col)"), index (col) #4=3 ("index (col)")) -> (element #1=w269:dbl[], element #2=w268:dbl[], element #3=w267:dbl[], element #4=w266:dbl[])  [unwired: 4 in]
              n122 = Bundle(w264, w269) -> (w265:cluster{dbl[], dbl[]})  [unwired: 1 in]
              n123 = Bundle(w264, w268) -> (w255:cluster{dbl[], dbl[]})  [unwired: 1 in]
              n124 = Bundle(w264, w267) -> (w263:cluster{dbl[], dbl[]})  [unwired: 1 in]
              n125 = Bundle(w264, w266) -> (w262:cluster{dbl[], dbl[]})  [unwired: 1 in]
              n126 = Build Array(w265, w255) -> (w259:cluster{dbl[], dbl[]}[])
              n127 = Build Array(w255) -> (w256:cluster{dbl[], dbl[]}[])
              n128 = Build Array(w263) -> (w257:cluster{dbl[], dbl[]}[])
              n129 = Build Array(w262) -> (w258:cluster{dbl[], dbl[]}[])
              n130 = local write "ROI Plot 01"(w259) -> ()
              n131 = local write "ROI Plot 02"(w256) -> ()
              n132 = local write "ROI Plot 03"(w257) -> ()
              n133 = local write "ROI Plot 04"(w258) -> ()
            }
          }
        }
      }
      event "Position (µm)": Value Change {
        n134 = event-data() -> ("NewVal"=w302:dbl)  [unwired: 1 in]
        n135 = Build Array(w302) -> (w301:dbl[])
        n136 = call "Stages Messenger.vi"("Stage Notifier Name"=w303, "Actions"=Stage_Actions."MOVE", "Setpoint"=w301, "Exit While Busy?"=TRUE) -> ()  [unwired: 8 in, 4 out]
      }
      event "Velocity (µm/s)": Value Change {
        n137 = event-data() -> ("NewVal"=w306:dbl)  [unwired: 1 in]
        n138 = call "Stages Messenger.vi"("Stage Notifier Name"=w311, "Actions"=Stage_Actions."VELOCITY", "Velocity"=w306) -> ()  [unwired: 9 in, 4 out]
      }
      event "Initial Guess Image 01", "Initial Guess Image 02", "Initial Guess Image 03", "Initial Guess Image 04": Value Change {
        n139 = event-data() -> ("CtlRef"=w316:refnum<vi>, "NewVal"=w318:T1)  [unwired: 1 in]
        n140 = property class="Clust (strict)"(reference=w316) -> ("Label.Text"=w314:string)  [unwired: 1 in, 2 out]
        n141 = case shown="\"Initial Guess Image 01\"" w314 {
          tunnel: w318 -> [_ w320 w369 w401 w433]
          tunnel: w317 -> [_ w325 w357 w389 w421]
          tunnel: w315 -> [_ w324 w356 w388 w420]
          tunnel: w315 -> [_ w321 w353 w385 w417]
          frame Default {
          }
          frame "Initial Guess Image 01" {
            w335 = 1000.0 ("Number of Points")
            n142 = Unbundle By Name(w320) -> ("Offset"=w332:dbl, "Amplitude"=w331:dbl, "Wavelength"=w330:dbl, "Phase"=w329:dbl)
            n143 = Array Max & Min(array=w321) -> (max value=w323:dbl, min value=w322:dbl)  [unwired: 2 out]
            n144 = Subtract(x=w323, y=w322) -> (x-y=w333:dbl)
            n145 = Divide(x=w333, y=w335) -> (x/y=w334:dbl)
            n146 = To Long Integer(number=w335) -> (32bit integer=w336:i32)
            n147 = for {
              N: w336 -> [_]
              tunnel: w334 -> [w350]
              tunnel: [w348] -> w328 mode=indexing
              tunnel: w322 -> [w343]
              tunnel: w332 -> [w347]
              tunnel: w331 -> [w346]
              tunnel: w330 -> [w345]
              tunnel: w329 -> [w344]
              tunnel: [w342] -> w327 mode=indexing
              i -> [w352]
              n148 = To Double Precision Float(number=w352) -> (double precision float=w351:dbl)
              n149 = Multiply(x=w350, y=w351) -> (x*y=w349:dbl)
              n150 = Add(x=w349, y=w343) -> (x+y=w342:dbl)
              n151 = formula code="y=y0+a*sin(((2*pi/w)*x)+p);"("w"=w345, "y0"=w347, "a"=w346, "p"=w344, "x"=w342, "pi"=3.141592653589793) -> ("y"=w348:dbl)
            }
            n152 = Index Array(array=w325, index (col)=0 ("disabled index (col)")) -> (element=w339:dbl[])  [unwired: 1 in]
            n153 = Bundle(w327, w328) -> (w326:cluster{dbl[], dbl[]})  [unwired: 1 in]
            n154 = Bundle("array"=w324, "array"=w339) -> (w338:cluster{"array":dbl[], "array":dbl[]})  [unwired: 1 in]
            n155 = Build Array(w338, w326) -> (w337:cluster{"array":dbl[], "array":dbl[]}[])
            n156 = local write "ROI Plot 01"(w337) -> ()
          }
          frame "Initial Guess Image 02" {
            w367 = 1000.0 ("Number of Points")
            n157 = Unbundle By Name(w369) -> ("Offset"=w364:dbl, "Amplitude"=w363:dbl, "Wavelength"=w362:dbl, "Phase"=w361:dbl)
            n158 = Array Max & Min(array=w353) -> (max value=w355:dbl, min value=w354:dbl)  [unwired: 2 out]
            n159 = Subtract(x=w355, y=w354) -> (x-y=w365:dbl)
            n160 = Divide(x=w365, y=w367) -> (x/y=w366:dbl)
            n161 = To Long Integer(number=w367) -> (32bit integer=w368:i32)
            n162 = for {
              N: w368 -> [_]
              tunnel: w366 -> [w382]
              tunnel: [w380] -> w360 mode=indexing
              tunnel: w354 -> [w375]
              tunnel: w364 -> [w379]
              tunnel: w363 -> [w378]
              tunnel: w362 -> [w377]
              tunnel: w361 -> [w376]
              tunnel: [w374] -> w359 mode=indexing
              i -> [w384]
              n163 = To Double Precision Float(number=w384) -> (double precision float=w383:dbl)
              n164 = Multiply(x=w382, y=w383) -> (x*y=w381:dbl)
              n165 = Add(x=w381, y=w375) -> (x+y=w374:dbl)
              n166 = formula code="y=y0+a*sin(((2*3.1415/w)*x)+p);"("w"=w377, "y0"=w379, "a"=w378, "p"=w376, "x"=w374) -> ("y"=w380:dbl)
            }
            n167 = Index Array(array=w357, index (col)=1 ("disabled index (col)")) -> (element=w372:dbl[])  [unwired: 1 in]
            n168 = Bundle(w359, w360) -> (w358:cluster{dbl[], dbl[]})  [unwired: 1 in]
            n169 = Bundle("array"=w356, "array"=w372) -> (w371:cluster{"array":dbl[], "array":dbl[]})  [unwired: 1 in]
            n170 = Build Array(w371, w358) -> (w370:cluster{"array":dbl[], "array":dbl[]}[])
            n171 = local write "ROI Plot 02"(w370) -> ()
          }
          frame "Initial Guess Image 03" {
            w399 = 1000.0 ("Number of Points")
            n172 = Unbundle By Name(w401) -> ("Offset"=w396:dbl, "Amplitude"=w395:dbl, "Wavelength"=w394:dbl, "Phase"=w393:dbl)
            n173 = Array Max & Min(array=w385) -> (max value=w387:dbl, min value=w386:dbl)  [unwired: 2 out]
            n174 = Subtract(x=w387, y=w386) -> (x-y=w397:dbl)
            n175 = Divide(x=w397, y=w399) -> (x/y=w398:dbl)
            n176 = To Long Integer(number=w399) -> (32bit integer=w400:i32)
            n177 = for {
              N: w400 -> [_]
              tunnel: w398 -> [w414]
              tunnel: [w412] -> w392 mode=indexing
              tunnel: w386 -> [w407]
              tunnel: w396 -> [w411]
              tunnel: w395 -> [w410]
              tunnel: w394 -> [w409]
              tunnel: w393 -> [w408]
              tunnel: [w406] -> w391 mode=indexing
              i -> [w416]
              n178 = To Double Precision Float(number=w416) -> (double precision float=w415:dbl)
              n179 = Multiply(x=w414, y=w415) -> (x*y=w413:dbl)
              n180 = Add(x=w413, y=w407) -> (x+y=w406:dbl)
              n181 = formula code="y=y0+a*sin(((2*3.1415/w)*x)+p);"("w"=w409, "y0"=w411, "a"=w410, "p"=w408, "x"=w406) -> ("y"=w412:dbl)
            }
            n182 = Index Array(array=w389, index (col)=2 ("disabled index (col)")) -> (element=w404:dbl[])  [unwired: 1 in]
            n183 = Bundle(w391, w392) -> (w390:cluster{dbl[], dbl[]})  [unwired: 1 in]
            n184 = Bundle("array"=w388, "array"=w404) -> (w403:cluster{"array":dbl[], "array":dbl[]})  [unwired: 1 in]
            n185 = Build Array(w403, w390) -> (w402:cluster{"array":dbl[], "array":dbl[]}[])
            n186 = local write "ROI Plot 03"(w402) -> ()
          }
          frame "Initial Guess Image 04" {
            w431 = 1000.0 ("Number of Points")
            n187 = Unbundle By Name(w433) -> ("Offset"=w428:dbl, "Amplitude"=w427:dbl, "Wavelength"=w426:dbl, "Phase"=w425:dbl)
            n188 = Array Max & Min(array=w417) -> (max value=w419:dbl, min value=w418:dbl)  [unwired: 2 out]
            n189 = Subtract(x=w419, y=w418) -> (x-y=w429:dbl)
            n190 = Divide(x=w429, y=w431) -> (x/y=w430:dbl)
            n191 = To Long Integer(number=w431) -> (32bit integer=w432:i32)
            n192 = for {
              N: w432 -> [_]
              tunnel: w430 -> [w446]
              tunnel: [w444] -> w424 mode=indexing
              tunnel: w418 -> [w439]
              tunnel: w428 -> [w443]
              tunnel: w427 -> [w442]
              tunnel: w426 -> [w441]
              tunnel: w425 -> [w440]
              tunnel: [w438] -> w423 mode=indexing
              i -> [w448]
              n193 = To Double Precision Float(number=w448) -> (double precision float=w447:dbl)
              n194 = Multiply(x=w446, y=w447) -> (x*y=w445:dbl)
              n195 = Add(x=w445, y=w439) -> (x+y=w438:dbl)
              n196 = formula code="y=y0+a*sin(((2*3.1415/w)*x)+p);"("w"=w441, "y0"=w443, "a"=w442, "p"=w440, "x"=w438) -> ("y"=w444:dbl)
            }
            n197 = Index Array(array=w421, index (col)=3 ("disabled index (col)")) -> (element=w436:dbl[])  [unwired: 1 in]
            n198 = Bundle(w423, w424) -> (w422:cluster{dbl[], dbl[]})  [unwired: 1 in]
            n199 = Bundle("array"=w420, "array"=w436) -> (w435:cluster{"array":dbl[], "array":dbl[]})  [unwired: 1 in]
            n200 = Build Array(w435, w422) -> (w434:cluster{"array":dbl[], "array":dbl[]}[])
            n201 = local write "ROI Plot 04"(w434) -> ()
          }
        }
      }
      event "Fit 01", "Fit 02", "Fit 03", "Fit 04": Value Change {
        n202 = event-data() -> ("CtlRef"=w454:refnum<vi>)  [unwired: 1 in, 1 out]
        n203 = property class="Bool"(reference=w454) -> ("Label.Text"=w453:string)  [unwired: 1 in, 2 out]
        n204 = case shown="\"Fit 01\"" w453 {
          tunnel: T11 {"model"="y0+a*sin(((2*3.1415/w)*x)+p)", "Parameters"=["y0", "a", "w", "p"], "x"="x"} ("model description") -> [_ w484 w528 w572 w616]
          tunnel: w451 -> [_ w488 w532 w576 w620]
          tunnel: w450 -> [_ w485 w529 w573 w617]
          tunnel: w451 -> [_ w468 w512 w556 w600]
          tunnel: w450 -> [_ w467 w511 w555 w599]
          tunnel: w450 -> [_ w462 w506 w550 w594]
          frame Default {
          }
          frame "Fit 01" {
            w474 = 1000.0 ("Number of Points")
            n205 = Index Array(array=w488, index (col)=0 ("disabled index (col)")) -> (element=w486:dbl[])  [unwired: 1 in]
            n206 = local read "Initial Guess Image 01"() -> (w483:T1)
            n207 = Cluster To Array(cluster=w483) -> (array=w482:dbl[])
            n208 = call-poly <vilib>:"Nonlinear Curve Fit.vi"("Y"=w486, "initial parameters"=w482, "X"=w485, "model description"=w484) -> ("best fit parameters"=w461:dbl[])  [unwired: 7 in, 4 out]
            n209 = Index Array(array=w461, index #1=0 ("index"), index #2=1 ("index"), index #3=2 ("index"), index #4=3 ("index")) -> (element #1=w460:dbl, element #2=w459:dbl, element #3=w458:dbl, element #4=w457:dbl)
            n210 = Array Max & Min(array=w462) -> (max value=w480:dbl, min value=w481:dbl)  [unwired: 2 out]
            n211 = Subtract(x=w480, y=w481) -> (x-y=w476:dbl)
            n212 = Bundle("Numeric"=w460, "Numeric"=w459, "Numeric"=w458, "Numeric"=w457) -> (w456:T13)  [unwired: 1 in]
            n213 = Divide(x=w476, y=w474) -> (x/y=w475:dbl)
            n214 = To Long Integer(number=w474) -> (32bit integer=w473:i32)
            n215 = local write "Initial Guess Image 01"(w456) -> ()
            n216 = for {
              N: w473 -> [_]
              tunnel: w475 -> [w497]
              tunnel: [w495] -> w477 mode=indexing
              tunnel: w481 -> [w490]
              tunnel: w460 -> [w494]
              tunnel: w459 -> [w493]
              tunnel: w458 -> [w492]
              tunnel: w457 -> [w491]
              tunnel: [w489] -> w478 mode=indexing
              i -> [w499]
              n217 = To Double Precision Float(number=w499) -> (double precision float=w498:dbl)
              n218 = Multiply(x=w497, y=w498) -> (x*y=w496:dbl)
              n219 = Add(x=w496, y=w490) -> (x+y=w489:dbl)
              n220 = formula code="y=y0+a*sin(((2*3.1415/w)*x)+p);"("w"=w492, "y0"=w494, "a"=w493, "p"=w491, "x"=w489) -> ("y"=w495:dbl)
            }
            n221 = Index Array(array=w468, index (col)=0 ("disabled index (col)")) -> (element=w470:dbl[])  [unwired: 1 in]
            n222 = Bundle(w478, w477) -> (w479:cluster{dbl[], dbl[]})  [unwired: 1 in]
            n223 = Bundle("array"=w467, "array"=w470) -> (w471:cluster{"array":dbl[], "array":dbl[]})  [unwired: 1 in]
            n224 = Build Array(w471, w479) -> (w472:cluster{"array":dbl[], "array":dbl[]}[])
            n225 = local write "ROI Plot 01"(w472) -> ()
          }
          frame "Fit 02" {
            w518 = 1000.0 ("Number of Points")
            n226 = Index Array(array=w532, index (col)=1 ("disabled index (col)")) -> (element=w530:dbl[])  [unwired: 1 in]
            n227 = local read "Initial Guess Image 02"() -> (w527:T1)
            n228 = Cluster To Array(cluster=w527) -> (array=w526:dbl[])
            n229 = call-poly <vilib>:"Nonlinear Curve Fit.vi"("Y"=w530, "initial parameters"=w526, "X"=w529, "model description"=w528) -> ("best fit parameters"=w505:dbl[])  [unwired: 7 in, 4 out]
            n230 = Index Array(array=w505, index #1=0 ("index"), index #2=1 ("index"), index #3=2 ("index"), index #4=3 ("index")) -> (element #1=w504:dbl, element #2=w503:dbl, element #3=w502:dbl, element #4=w501:dbl)
            n231 = Array Max & Min(array=w506) -> (max value=w524:dbl, min value=w525:dbl)  [unwired: 2 out]
            n232 = Subtract(x=w524, y=w525) -> (x-y=w520:dbl)
            n233 = Bundle("Numeric"=w504, "Numeric"=w503, "Numeric"=w502, "Numeric"=w501) -> (w500:T13)  [unwired: 1 in]
            n234 = Divide(x=w520, y=w518) -> (x/y=w519:dbl)
            n235 = To Long Integer(number=w518) -> (32bit integer=w517:i32)
            n236 = local write "Initial Guess Image 02"(w500) -> ()
            n237 = for {
              N: w517 -> [_]
              tunnel: w519 -> [w541]
              tunnel: [w539] -> w521 mode=indexing
              tunnel: w525 -> [w534]
              tunnel: w504 -> [w538]
              tunnel: w503 -> [w537]
              tunnel: w502 -> [w536]
              tunnel: w501 -> [w535]
              tunnel: [w533] -> w522 mode=indexing
              i -> [w543]
              n238 = To Double Precision Float(number=w543) -> (double precision float=w542:dbl)
              n239 = Multiply(x=w541, y=w542) -> (x*y=w540:dbl)
              n240 = Add(x=w540, y=w534) -> (x+y=w533:dbl)
              n241 = formula code="y=y0+a*sin(((2*3.1415/w)*x)+p);"("w"=w536, "y0"=w538, "a"=w537, "p"=w535, "x"=w533) -> ("y"=w539:dbl)
            }
            n242 = Index Array(array=w512, index (col)=1 ("disabled index (col)")) -> (element=w514:dbl[])  [unwired: 1 in]
            n243 = Bundle(w522, w521) -> (w523:cluster{dbl[], dbl[]})  [unwired: 1 in]
            n244 = Bundle("array"=w511, "array"=w514) -> (w515:cluster{"array":dbl[], "array":dbl[]})  [unwired: 1 in]
            n245 = Build Array(w515, w523) -> (w516:cluster{"array":dbl[], "array":dbl[]}[])
            n246 = local write "ROI Plot 02"(w516) -> ()
          }
          frame "Fit 03" {
            w562 = 1000.0 ("Number of Points")
            n247 = Index Array(array=w576, index (col)=2 ("disabled index (col)")) -> (element=w574:dbl[])  [unwired: 1 in]
            n248 = local read "Initial Guess Image 03"() -> (w571:T1)
            n249 = Cluster To Array(cluster=w571) -> (array=w570:dbl[])
            n250 = call-poly <vilib>:"Nonlinear Curve Fit.vi"("Y"=w574, "initial parameters"=w570, "X"=w573, "model description"=w572) -> ("best fit parameters"=w549:dbl[])  [unwired: 7 in, 4 out]
            n251 = Index Array(array=w549, index #1=0 ("index"), index #2=1 ("index"), index #3=2 ("index"), index #4=3 ("index")) -> (element #1=w548:dbl, element #2=w547:dbl, element #3=w546:dbl, element #4=w545:dbl)
            n252 = Array Max & Min(array=w550) -> (max value=w568:dbl, min value=w569:dbl)  [unwired: 2 out]
            n253 = Subtract(x=w568, y=w569) -> (x-y=w564:dbl)
            n254 = Bundle("Numeric"=w548, "Numeric"=w547, "Numeric"=w546, "Numeric"=w545) -> (w544:T13)  [unwired: 1 in]
            n255 = Divide(x=w564, y=w562) -> (x/y=w563:dbl)
            n256 = To Long Integer(number=w562) -> (32bit integer=w561:i32)
            n257 = local write "Initial Guess Image 03"(w544) -> ()
            n258 = for {
              N: w561 -> [_]
              tunnel: w563 -> [w585]
              tunnel: [w583] -> w565 mode=indexing
              tunnel: w569 -> [w578]
              tunnel: w548 -> [w582]
              tunnel: w547 -> [w581]
              tunnel: w546 -> [w580]
              tunnel: w545 -> [w579]
              tunnel: [w577] -> w566 mode=indexing
              i -> [w587]
              n259 = To Double Precision Float(number=w587) -> (double precision float=w586:dbl)
              n260 = Multiply(x=w585, y=w586) -> (x*y=w584:dbl)
              n261 = Add(x=w584, y=w578) -> (x+y=w577:dbl)
              n262 = formula code="y=y0+a*sin(((2*3.1415/w)*x)+p);"("w"=w580, "y0"=w582, "a"=w581, "p"=w579, "x"=w577) -> ("y"=w583:dbl)
            }
            n263 = Index Array(array=w556, index (col)=2 ("disabled index (col)")) -> (element=w558:dbl[])  [unwired: 1 in]
            n264 = Bundle(w566, w565) -> (w567:cluster{dbl[], dbl[]})  [unwired: 1 in]
            n265 = Bundle("array"=w555, "array"=w558) -> (w559:cluster{"array":dbl[], "array":dbl[]})  [unwired: 1 in]
            n266 = Build Array(w559, w567) -> (w560:cluster{"array":dbl[], "array":dbl[]}[])
            n267 = local write "ROI Plot 03"(w560) -> ()
          }
          frame "Fit 04" {
            w606 = 1000.0 ("Number of Points")
            n268 = Index Array(array=w620, index (col)=3 ("disabled index (col)")) -> (element=w618:dbl[])  [unwired: 1 in]
            n269 = local read "Initial Guess Image 04"() -> (w615:T1)
            n270 = Cluster To Array(cluster=w615) -> (array=w614:dbl[])
            n271 = call-poly <vilib>:"Nonlinear Curve Fit.vi"("Y"=w618, "initial parameters"=w614, "X"=w617, "model description"=w616) -> ("best fit parameters"=w593:dbl[])  [unwired: 7 in, 4 out]
            n272 = Index Array(array=w593, index #1=0 ("index"), index #2=1 ("index"), index #3=2 ("index"), index #4=3 ("index")) -> (element #1=w592:dbl, element #2=w591:dbl, element #3=w590:dbl, element #4=w589:dbl)
            n273 = Array Max & Min(array=w594) -> (max value=w612:dbl, min value=w613:dbl)  [unwired: 2 out]
            n274 = Subtract(x=w612, y=w613) -> (x-y=w608:dbl)
            n275 = Bundle("Numeric"=w592, "Numeric"=w591, "Numeric"=w590, "Numeric"=w589) -> (w588:T13)  [unwired: 1 in]
            n276 = Divide(x=w608, y=w606) -> (x/y=w607:dbl)
            n277 = To Long Integer(number=w606) -> (32bit integer=w605:i32)
            n278 = local write "Initial Guess Image 04"(w588) -> ()
            n279 = for {
              N: w605 -> [_]
              tunnel: w607 -> [w629]
              tunnel: [w627] -> w609 mode=indexing
              tunnel: w613 -> [w622]
              tunnel: w592 -> [w626]
              tunnel: w591 -> [w625]
              tunnel: w590 -> [w624]
              tunnel: w589 -> [w623]
              tunnel: [w621] -> w610 mode=indexing
              i -> [w631]
              n280 = To Double Precision Float(number=w631) -> (double precision float=w630:dbl)
              n281 = Multiply(x=w629, y=w630) -> (x*y=w628:dbl)
              n282 = Add(x=w628, y=w622) -> (x+y=w621:dbl)
              n283 = formula code="y=y0+a*sin(((2*3.1415/w)*x)+p);"("w"=w624, "y0"=w626, "a"=w625, "p"=w623, "x"=w621) -> ("y"=w627:dbl)
            }
            n284 = Index Array(array=w600, index (col)=3 ("disabled index (col)")) -> (element=w602:dbl[])  [unwired: 1 in]
            n285 = Bundle(w610, w609) -> (w611:cluster{dbl[], dbl[]})  [unwired: 1 in]
            n286 = Bundle("array"=w599, "array"=w602) -> (w603:cluster{"array":dbl[], "array":dbl[]})  [unwired: 1 in]
            n287 = Build Array(w603, w611) -> (w604:cluster{"array":dbl[], "array":dbl[]}[])
            n288 = local write "ROI Plot 04"(w604) -> ()
          }
        }
      }
      event "Save Data": Value Change {
        n289 = event-data() -> ()  [unwired: 1 in, 6 out]
        n290 = Transpose 2D Array(2D array=w636) -> (transposed array=w635:dbl[][])
        n291 = Build Array (concatenate)(w634, w635) -> (w633:dbl[][])
        n292 = Transpose 2D Array(2D array=w633) -> (transposed array=w632:dbl[][])
        n293 = call-poly <vilib>:"Write Delimited Spreadsheet.vi"("2D data"=w632) -> ()  [unwired: 13 in, 2 out]
      }
      event "Overlay Plot": Value Change {
        n294 = event-data() -> ()  [unwired: 1 in, 6 out]
        n295 = Index Array(array=w647, index (col) #1=0 ("disabled index (col)"), index (col) #2=1 ("index (col)")) -> (element #1=w643:dbl[], element #2=w642:dbl[])  [unwired: 2 in]
        n296 = Bundle("array"=w644, "array"=w642) -> (w640:cluster{"array":dbl[], "array":dbl[]})  [unwired: 1 in]
        n297 = Bundle("array"=w644, "array"=w643) -> (w641:cluster{"array":dbl[], "array":dbl[]})  [unwired: 1 in]
        n298 = Build Array(w641, w640) -> (→"Overlay Plot Graph":cluster{"array":dbl[], "array":dbl[]}[])
      }
      event "Quit": Value Change {
        n299 = event-data() -> ("NewVal"=w653:bool)  [unwired: 1 in]
        n300 = Release Notifier(notifier=w655) -> ()  [unwired: 2 in, 3 out]
        n301 = call "IMAQ Dispose"("Image"=w654) -> ()  [unwired: 5 in, 1 out]
      }
    }
  }
  n302 = local write "Quit"(w22) -> ()
